vi "NanoRoute3D.vi"(2 "Incoming Handle":i32) -> ()   [LabVIEW 2012]
uses:
  <vilib>/Utility/inputDevices.llb/keyboardAcquire.vi
  Madlib.dll
panel:
  out "fit graph once":bool
  out "Type Descriptor":i16[](array[numeric])
  out "Saved Route":T1
  in  "Tab Control":T2(tab)
  in  "include 6":bool=TRUE
  in  "include 5":bool=TRUE
  in  "include 4":bool=TRUE
  in  "include 3":bool=TRUE
  in  "include 2":bool=TRUE
  in  "include 1":bool=TRUE
  in  "stop":bool
  out "Firmware Profile":i16
  out "Firmware Version 2":i16
  out "Product ID (in hex) 2":string
  out "DAC resolution (bits)":i16
  out "ADC resolution (bits)":i16
  out "Dll Version":i16
  out "Dll Revision":i16
  out "ADC Freq (ms)":dbl format="%.4f"
  out "DAC Freq (ms)":dbl format="%.4f"
  out "X axis":bool
  out "Y axis":bool
  out "Z axis":bool
  out "Aux axis":bool
  out "X Calibration 2":dbl caption="Calibration (um)" format="%.3f"
  out "Y Calibration 2":dbl format="%.3f"
  out "Z Calibration 2":dbl format="%.3f"
  out "Aux Calibration 2":dbl format="%.3f"
  out "Serial # 2":i32
  in  "handleIndex":i32(ring)
  out "DeviceLoaded":bool
  in  "include 7":bool
  in  "include 8":bool
  in  "include 9":bool
  in  "include 10":bool
  in  "Remove All":bool
  in  "Set All":bool
  in  "SaveDeviceData":bool
  out "Device Data":string
  in  "Initialize/Release USB":bool
  in  "include 11":bool=TRUE
  in  "include 12":bool=TRUE
  in  "include 13":bool=TRUE
  in  "include 14":bool=TRUE
  in  "Run backwards":bool
  in  "Relative Start":bool
  in  "gamepad":bool
  out "LivePosition":enum32{"disable", "enable"}(tab)
  out "X-Axis":dbl format="%.4f"
  out "Y-Axis":dbl format="%.4f"
  out "Z-Axis":dbl format="%.4f"
  in  "Command X":bool
  in  "Command Y":bool
  in  "Command Z":bool
  in  "X command":dbl format="%#.4f"
  in  "Z command":dbl format="%#_4f"
  in  "Y command":dbl format="%#.4f"
  out "Scanning Indicator":bool
  in  "LivePosition":bool
  in  "um":dbl
  in  "(ms)":dbl=100.0 min=0.033
  in  "Path Units":u8(ring) items=["ms", "dpts"]
  in  "Load":bool
  in  "SAVE":bool
  out "Custom Scans":T3(tab)
  in  "Pixel dwell":u32
  in  "Begin Raster":bool
  in  "Pixel":u32(ring)=1 items=["X axis"=1, "Y axis"=2, "Z axis"=3]
  in  "Line":u32(ring)=2 items=["X axis"=1, "Y axis"=2, "Z axis"=3, "Do Nothing"=4]
  in  "Frame":u32(ring)=3 items=["X axis"=1, "Y axis"=2, "Z axis"=3, "Do Nothing"=4]
  in  "Pixel delay":u32
  in  "End of Line delay":u32
  in  "Frame delay":u32
  out "Est. R.S. time":dbl format="%<%H:%M:%S>t"
  in  "Mirror motion on return?":bool=TRUE
  in  "Start of Line delay":u32
  in  "RaScAdvanced":bool
  out "Custom.name 2":string
  out "Custom.name 3":string
  in  "Ignore":bool
  in  "A/D Rate\n16-bit":dbl=2.0 min=0.033
  in  "A/D Rate\n20-bit":dbl(ring)=1.0 items=[".267ms"=0.267, ".5ms"=0.5, "1ms"=1.0, "2ms"=2.0, "10ms"=10.0, "17ms"=17.0, "20ms"=20.0]
  in  "Template":u16(ring) items=["Standard", "Single Axis Scan", "Multi-Axis Scan", "Raster Scan", "Custom Scan 1", "Custom Scan 2"]
  in  "Clear Graph":bool
  in  "WF\nAcq.":bool=TRUE
  in  "Run All Routes":bool
  out "Paths in Z Route:":u16
  out "Paths in Y Route:":u16
  in  "Axis":u32(ring)=1 items=["X axis"=1, "Y axis"=2, "Z axis"=3]
  out "Points in Route":i32
  out "Points in Current Path":i32
  in  "function:":string="sin(x)"
  out "Time to Command Route (ms):":dbl
  in  "Load Route":bool
  in  "Save Route":bool
  out "Paths in X Route:":u16
  in  "Reset":bool
  in  "Run Route":bool
  in  "Current #:":u16
  in  "DeletePath":bool
  in  "AddPath":bool
  in  "PrevPoint":bool
  in  "NextPoint":bool
  in  "Path Type":u16(ring) items=["Remain at", "Ramp to", "Apply Point Func:", "Apply Time Func:", "Custom Path 1", "Custom Path 2"]
  in  "offset":dbl[](array[numeric])
  out "Route Graph":cluster{dbl[], dbl[]}[](graph)=[{[0.0], [0.0]}, {[0.0, 1.0, 2.0, 3.0, 4.0, 5.0, 6.0, 7.0, 8.0, 9.0, 10.0, 11.0, 12.0, 13.0, 14.0, 15.0, 16.0, 17.0, 18.0, 19.0, 20.0, 21.0, 22.0, 23.0, 24.0, 25.0, 26.0, 27.0, 28.0, 29.0, 30.0, 31.0, 32.0, 33.0, 34.0, 35.0, 36.0, 37.0, 38.0, 39.0, 40.0, 41.0, 42.0, 43.0, 44.0, 45.0, 46.0, 47.0, 48.0, 49.0], [0.0, 0.0, 0.0, 0.0, 0.0, 0.0, 0.0, 0.0, 0.0, 0.0, 0.0, 0.0, 0.0, 0.0, 0.0, 0.0, 0.0, 0.0, 0.0, 0.0, 0.0, 0.0, 0.0, 0.0, 0.0, 0.0, 0.0, 0.0, 0.0, 0.0, 0.0, 0.0, 0.0, 0.0, 0.0, 0.0, 0.0, 0.0, 0.0, 0.0, 0.0, 0.0, 0.0, 0.0, 0.0, 0.0, 0.0, 0.0, 0.0, 0.0]}, {[], []}, {[], []}, {[], []}, {[], []}, {[], []}]
  in  "View Start of Scan ISS Commands":bool caption="View End of Scan ISS Commands"
  in  "Adv ISS Control":bool
  out "ISS pre-post config.":enum32{"Basic", "Adv. Start", "Adv. End"}(tab)
  in  "Start:Pixel":bool
  in  "Start:Line":bool
  in  "Start:Frame":bool
  in  "Start:Aux":bool
  in  "End:Pixel":bool
  in  "End:Line":bool
  in  "End:Frame":bool
  in  "End:Aux":bool
  in  "Start:Pixel:Order":enum16{"1st", "2nd", "3rd", "4th"}(ring)
  in  "Start:Line:Order":enum16{"1st", "2nd", "3rd", "4th"}(ring)=enum."2nd"
  in  "Start:Frame:Order":enum16{"1st", "2nd", "3rd", "4th"}(ring)=enum."3rd"
  in  "Start:Aux:Order":enum16{"1st", "2nd", "3rd", "4th"}(ring)=enum."4th"
  in  "End:Pixel:Order":enum16{"1st", "2nd", "3rd", "4th"}(ring)
  in  "End:Line:Order":enum16{"1st", "2nd", "3rd", "4th"}(ring)=enum."2nd"
  in  "End:Frame:Order":enum16{"1st", "2nd", "3rd", "4th"}(ring)=enum."3rd"
  in  "End:Aux:Order":enum16{"1st", "2nd", "3rd", "4th"}(ring)=enum."4th"
  out "ISSAdv Start":dbl
  in  "AuxStartAdv 11":bool=TRUE
  in  "AuxStartAdv 10":bool=TRUE
  in  "AuxStartAdv 9":bool=TRUE
  in  "AuxStartAdv 8":bool=TRUE
  in  "AuxStartAdv 7":bool=TRUE
  in  "AuxStartAdv 6":bool=TRUE
  in  "AuxStartAdv 5":bool=TRUE
  in  "AuxStartAdv 4":bool=TRUE
  in  "AuxStartAdv 3":bool=TRUE
  in  "AuxStartAdv 2":bool=TRUE
  in  "AuxStartAdv 1":bool=TRUE
  in  "FrameStartAdv 11":bool=TRUE
  in  "FrameStartAdv 10":bool=TRUE
  in  "FrameStartAdv 9":bool=TRUE
  in  "FrameStartAdv 8":bool=TRUE
  in  "FrameStartAdv 7":bool=TRUE
  in  "FrameStartAdv 6":bool=TRUE
  in  "FrameStartAdv 5":bool=TRUE
  in  "FrameStartAdv 4":bool=TRUE
  in  "FrameStartAdv 3":bool=TRUE
  in  "FrameStartAdv 2":bool=TRUE
  in  "FrameStartAdv 1":bool=TRUE
  in  "LineStartAdv 11":bool=TRUE
  in  "LineStartAdv 10":bool=TRUE
  in  "LineStartAdv 9":bool=TRUE
  in  "LineStartAdv 8":bool=TRUE
  in  "LineStartAdv 7":bool=TRUE
  in  "LineStartAdv 6":bool=TRUE
  in  "LineStartAdv 5":bool=TRUE
  in  "LineStartAdv 4":bool=TRUE
  in  "LineStartAdv 3":bool=TRUE
  in  "LineStartAdv 2":bool=TRUE
  in  "LineStartAdv 1":bool
  in  "PixStartAdv 11":bool=TRUE
  in  "PixStartAdv 10":bool=TRUE
  in  "PixStartAdv 9":bool=TRUE
  in  "PixStartAdv 8":bool=TRUE
  in  "PixStartAdv 7":bool=TRUE
  in  "PixStartAdv 6":bool=TRUE
  in  "PixStartAdv 5":bool=TRUE
  in  "PixStartAdv 4":bool=TRUE
  in  "PixStartAdv 3":bool=TRUE
  in  "PixStartAdv 2":bool=TRUE
  in  "PixStartAdv 1":bool=TRUE
  in  "ISS msStart 11":dbl
  in  "ISS msStart 10":dbl
  in  "ISS msStart 9":dbl
  in  "ISS msStart 8":dbl
  in  "ISS msStart 7":dbl
  in  "ISS msStart 6":dbl
  in  "ISS msStart 5":dbl
  in  "ISS msStart 4":dbl
  in  "ISS msStart 3":dbl
  in  "ISS msStart 2":dbl
  in  "ISS msStart 1":dbl
  in  "ISS msEnd 1":dbl
  in  "ISS msEnd 2":dbl
  in  "ISS msEnd 3":dbl
  in  "ISS msEnd 4":dbl
  in  "ISS msEnd 5":dbl
  in  "ISS msEnd 6":dbl
  in  "ISS msEnd 7":dbl
  in  "ISS msEnd 8":dbl
  in  "ISS msEnd 9":dbl
  in  "ISS msEnd 10":dbl
  in  "ISS msEnd 11":dbl
  in  "PixEndAdv 1":bool=TRUE
  in  "PixEndAdv 2":bool=TRUE
  in  "PixEndAdv 3":bool=TRUE
  in  "PixEndAdv 4":bool=TRUE
  in  "PixEndAdv 5":bool=TRUE
  in  "PixEndAdv 6":bool=TRUE
  in  "PixEndAdv 7":bool=TRUE
  in  "PixEndAdv 8":bool=TRUE
  in  "PixEndAdv 9":bool=TRUE
  in  "PixEndAdv 10":bool=TRUE
  in  "PixEndAdv 11":bool=TRUE
  in  "LineEndAdv 1":bool
  in  "LineEndAdv 2":bool=TRUE
  in  "LineEndAdv 3":bool=TRUE
  in  "LineEndAdv 4":bool=TRUE
  in  "LineEndAdv 5":bool=TRUE
  in  "LineEndAdv 6":bool=TRUE
  in  "LineEndAdv 7":bool=TRUE
  in  "LineEndAdv 8":bool=TRUE
  in  "LineEndAdv 9":bool=TRUE
  in  "LineEndAdv 10":bool=TRUE
  in  "LineEndAdv 11":bool=TRUE
  in  "FrameEndAdv 1":bool=TRUE
  in  "FrameEndAdv 2":bool=TRUE
  in  "FrameEndAdv 3":bool=TRUE
  in  "FrameEndAdv 4":bool=TRUE
  in  "FrameEndAdv 5":bool=TRUE
  in  "FrameEndAdv 6":bool=TRUE
  in  "FrameEndAdv 7":bool=TRUE
  in  "FrameEndAdv 8":bool=TRUE
  in  "FrameEndAdv 9":bool=TRUE
  in  "FrameEndAdv 10":bool=TRUE
  in  "FrameEndAdv 11":bool=TRUE
  in  "AuxEndAdv 1":bool=TRUE
  in  "AuxEndAdv 2":bool=TRUE
  in  "AuxEndAdv 3":bool=TRUE
  in  "AuxEndAdv 4":bool=TRUE
  in  "AuxEndAdv 5":bool=TRUE
  in  "AuxEndAdv 6":bool=TRUE
  in  "AuxEndAdv 7":bool=TRUE
  in  "AuxEndAdv 8":bool=TRUE
  in  "AuxEndAdv 9":bool=TRUE
  in  "AuxEndAdv 10":bool=TRUE
  in  "AuxEndAdv 11":bool=TRUE
  in  "PulseAux":bool
  in  "PulseFrame":bool
  in  "PulseLine":bool
  in  "LineRestore":bool
  in  "AuxRestore":bool
  in  "LinePol":enum16{"Low", "High"}(ring)
  in  "LinePulse":enum16{"Low to High", "High to Low"}(ring)
  in  "LineBindAxis":T4(ring)
  in  "FramePol":enum16{"Low", "High"}(ring)
  in  "FramePulse":enum16{"Low to High", "High to Low"}(ring)
  in  "FrameBindAxis":T4(ring)
  in  "FrameRestore":bool
  in  "AuxPol":enum16{"Low", "High"}(ring)
  in  "AuxPulse":enum16{"Low to High", "High to Low"}(ring)
  in  "AuxBindAxis":T4(ring)
  in  "PulsePix":bool
  in  "PixBindAxis":T4(ring)
  in  "PixPulse":enum16{"Low to High", "High to Low"}(ring)
  in  "ISSReset":bool
  in  "PixRestore":bool
  in  "ISSConfirm":bool
  in  "PixPol":enum16{"Low", "High"}(ring)
  in  "Export DAC":bool
  in  "Export ADC":bool
  in  "Now Showing":u32(ring) items=["Individual Route Scan", "Run All Routes Scan", "Raster Scan", "Custom 1", "Custom 2"]
  in  "Back Remove":u32(slide) step=1 scale=0.0..100.0
  in  "FrontRemove":u32(slide) step=1 scale=0.0..100.0
  in  "Y-Axis Display":u8(ring)=2 items=["Point by Point", "Time in milliseconds", "Axis: X Position", "Axis: Y Position", "Axis: Z Position"]
  in  "Legend Visible":bool
  in  "Interpolation?":bool=TRUE
  in  "Visible?":bool=TRUE
  in  "X-Axis Display":u8(ring) items=["Point by Point", "Time in milliseconds", "Axis: X Position", "Axis: Y Position", "Axis: Z Position"]
  in  "Active Plot":u32(ring) items=["ADC values (Sensor)", "DAC values (Command)"]
  out "Image Graph":cluster{dbl[], dbl[]}[](graph)
  # "Device Information"
  # "Version 2.01"
  # "Device Information"
  # "Data will be saved to a text file in the following format:"
  # "Load/Release USB(s)"
  # "Include/Disinclude All:"
  # "Available Devices:"
  # "Calibration (um)"
  # "Nano-Route  3D"
  # "®"
  # "VI State Control"
  # "Generate/Run Route"
  # "Scan Type"
  # "Device Settings"
  # "A/D\nRate"
  # "(ms)"
  # "New Path"
  # "over an interval of ..."
  # "dpts"
  # "Path Creation"
  # "Copy/Paste Route"
  # "Route Settings"
  # "Relative start"
  # "Nano-Drive Live Position"
  # "Gamepad"
  # "Check box at left to enable live position updates. This feature may interfere with your ISS settings"
  # "um"
  # "um"
  # "um"
  # "um"
  # "um"
  # "um"
  # "Raster Scan"
  # "ms"
  # "ms"
  # "ms"
  # "ms"
  # "ms"
  # "ISS Configuration"
  # "Pixel Clock"
  # "Line Clock"
  # "Frame Clock"
  # "Auxilary Clock"
  # "Polarity:"
  # "Polarity:"
  # "Polarity:"
  # "Polarity:"
  # "Pulse:"
  # "Pulse:"
  # "Pulse:"
  # "Pulse:"
  # "Bind Clock to Axis:"
  # "Bind Clock to Axis:"
  # "Bind Clock to Axis:"
  # "Bind Clock to Axis:"
  # "* Only one clock can be bound to an axis or event. Binding a second clock\n    replaces the first with the second (Nano-Route   3D prevents this action)."
  # "®"
  # "Confirm/Reset \nISS Configuration:"
  # "* Changes made here take no effect until confirmed."
  # "* Binding a Clock to an Axis will result in the suspension of \"Nano-Drive Live\n  Position\" reads."
  # "Programmatic ISS Control"
  # "Pulse Individual \nISS Clocks:"
  # "* Pulsing will reset Clock to Low polarity."
  # "Pulse clock before beginning each scan."
  # "Pulse clock at the end of each scan."
  # "Pixel clock"
  # "Pixel clock"
  # "Line clock"
  # "Line clock"
  # "Frame clock"
  # "Frame clock"
  # "Aux clock"
  # "Aux clock"
  # "milliseconds"
  # "ms"
  # "pixel clock"
  # "Start\nof \nScan"
  # "line clock"
  # "frame clock"
  # "aux clock"
  # "milliseconds"
  # "pixel clock"
  # "End\nof \nScan"
  # "line clock"
  # "frame clock"
  # "aux clock"
  # "Crop Data-\n Points From \n  Start/End"
  # "Plot to Edit:"
  # "X-Axis Repr.:"
  # "Graph Options"
  # "Plot Options"
  # "Now Showing:"
  # "Y-Axis Repr.:"
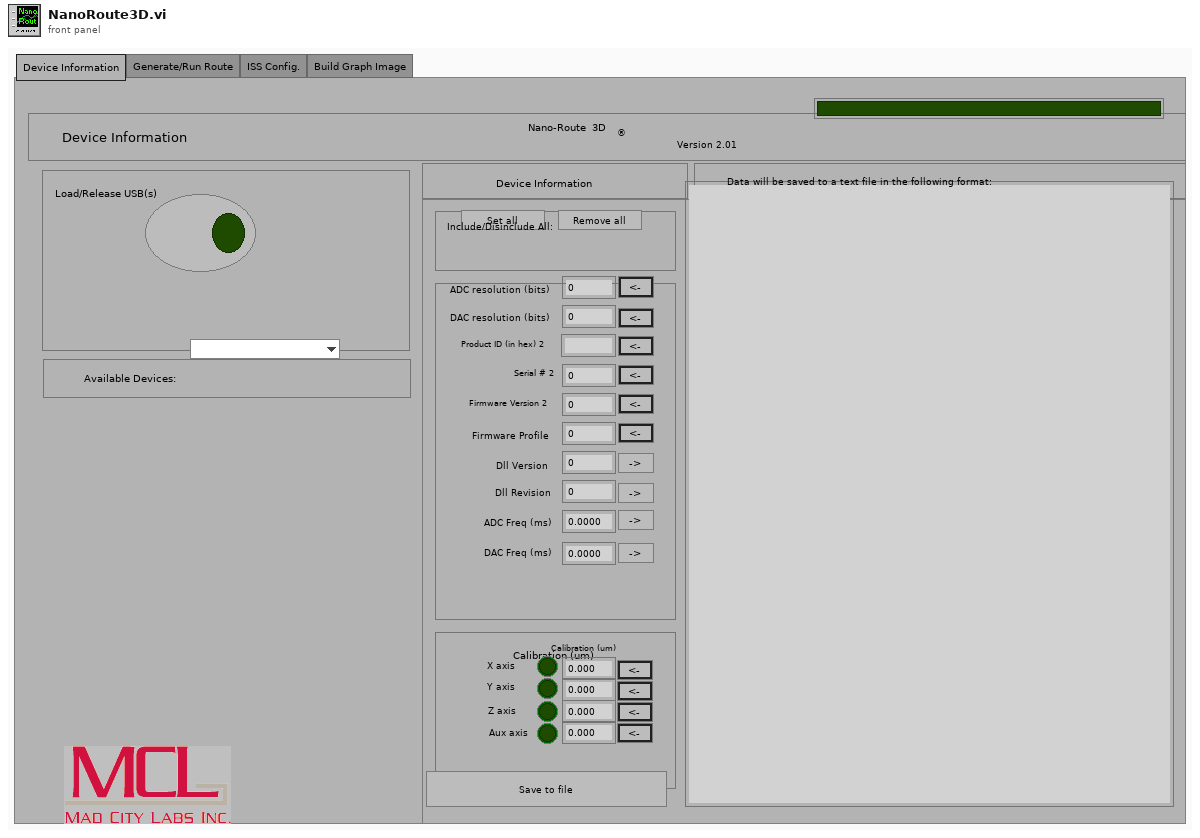
[diagram p1: front panel]
types:
  T1 = cluster{"t":cluster{dbl[], dbl[], i32[], u16[]}, "Current Path #:":u16, "# of Paths in Route:":u16}
  T2 = enum32{"Device Information", "Generate/Run Route", "ISS Config.", "Build Graph Image"}
  T3 = enum32{"Empty", "Raster Scan", "Custom 1", "Custom 2"}
  T4 = enum16{"Unbound", "X Axis", "Y Axis", "Z Axis", "Auxilary", "Waveform Read", "Waveform Write"}
  T5 = cluster{"Pixel delay":u32, "End of Line delay":u32, "Start of Line delay":u32, "Frame delay":u32, "Pixel dwell":u32}
  T6 = cluster{"X axis":bool, "Y axis":bool, "Z axis":bool}
  T7 = cluster{"Incoming Handle":i32, "Axis":u32, "A/D Rate\n16-bit 2":dbl}
  T8 = cluster{"RaSc16bitReadRate IN":dbl, "RaSc16bitWriteRate IN":dbl, "RaSc20bitWriteRate IN":dbl, "RaSc20bitReadRate IN":dbl, "Pixel uses Waveform Acquisition IN":bool, "RaSc16bit#ofReads IN":u32}
  T9 = cluster{"ISSReset":bool, "ISS Confirmed Options":cluster{"clock (1=Pixel)":i32, "Pixel Polarity":enum16{"Low", "High"}, "Pixel Pulse":enum16{"Low to High", "High to Low"}, "Pixel Bind":enum16{"Unbound", "X Axis", "Y Axis", "Z Axis", "Auxilary", "Waveform Read", "Waveform Write"}}, "ISS Confirmed Options":cluster{"clock (1=Pixel)":i32, "Pixel Polarity":enum16{"Low", "High"}, "Pixel Pulse":enum16{"Low to High", "High to Low"}, "Pixel Bind":enum16{"Unbound", "X Axis", "Y Axis", "Z Axis", "Auxilary", "Waveform Read", "Waveform Write"}}, "ISS Confirmed Options":cluster{"clock (1=Pixel)":i32, "Pixel Polarity":enum16{"Low", "High"}, "Pixel Pulse":enum16{"Low to High", "High to Low"}, "Pixel Bind":enum16{"Unbound", "X Axis", "Y Axis", "Z Axis", "Auxilary", "Waveform Read", "Waveform Write"}}, "ISS Confirmed Options":cluster{"clock (1=Pixel)":i32, "Pixel Polarity":enum16{"Low", "High"}, "Pixel Pulse":enum16{"Low to High", "High to Low"}, "Pixel Bind":enum16{"Unbound", "X Axis", "Y Axis", "Z Axis", "Auxilary", "Waveform Read", "Waveform Write"}}}
  T10 = cluster{"Custom 1 Read Arrays":cluster{"Z Read":cluster{dbl[], dbl[]}, "Y Read":cluster{i32[], dbl[]}, "Z Read":cluster{i32[], dbl[]}}, "Custom 1 Read Arrays":cluster{"Z Read":cluster{dbl[], dbl[]}, "Y Read":cluster{i32[], dbl[]}, "Z Read":cluster{i32[], dbl[]}}}
  T11 = cluster{"handlesListIndex":i32, "listOfHandlist":i32[], "sizeOfHandlesList":i32}
  T12 = cluster{"Read":cluster{dbl[], "Waveform Read":dbl[]}, "Read":cluster{dbl[], "Waveform Read":dbl[]}, "Read":cluster{dbl[], "Waveform Read":dbl[]}}
  T13 = enum16{"0", "1", "2", "3", "4", "5", "6", "7", "8", "9", "A", "B", "C", "D", "E", "F", "G", "H", "I", "J", "K", "L", "M", "N", "O", "P", "Q", "R", "S", "T", "U", "V", "W", "X", "Y", "Z", "F1", "F2", "F3", "F4", "F5", "F6", "F7", "F8", "F9", "F10", "F11", "F12", "F13", "F14", "F15", "ADD", "BACK", "BACKSLASH", "CAPITAL", "COMMA", "DECIMAL", "DELETE", "DIVIDE", "DOWN", "END", "EQUALS", "ESCAPE", "GRAVE (`)", "HOME", "INSERT", "LBRACKET", "LCONTROL", "LEFT", "L ALT", "LSHIFT", "LWIN", "MINUS", "MULTIPLY", "NEXT", "NUMLOCK", "NUMPAD_0", "NUMPAD_1", "NUMPAD_2", "NUMPAD_3", "NUMPAD_4", "NUMPAD_5", "NUMPAD_6", "NUMPAD_7", "NUMPAD_8", "NUMPAD_9", "PAUSE", "PERIOD", "PRIOR (PG UP)", "RBRACKET", "RCONTROL", "RETURN", "RIGHT", "R ALT", "RSHIFT", "RWIN", "SCROLL", "SEMICOLON", "SLASH", "SPACE", "SUBTRACT", "TAB", "UP", "ENTER (num pad)", "' (quote)"}[]
  T14 = cluster{cluster{dbl[], dbl[]}, cluster{dbl[], dbl[]}, cluster{dbl[], dbl[]}}
  T15 = cluster{string, cluster{"ADC resolution (bits)":i16, "DAC resolution (bits)":i16, "Product ID (in hex)":string, "Firmware Version":i16, "Firmware Profile":i16, "Dll Version":i16, "X axis":bool, "Y axis":bool, "Z axis":bool, "Aux axis":bool, "X Calibration":dbl, "Y Calibration":dbl, "Z Calibration":dbl, "Aux Calibration":dbl, "Dll Revision":i16, "ADC Freq (ms)":dbl, "DAC Freq (ms)":dbl, "Serial #":i32}, "X Calibration":dbl, "Y Calibration":dbl, "Z Calibration":dbl, bool}
  T16 = enum32{"Device Information", "Generate/Run Route", "ISS Config.", "Rptblty Test", "Build Graph Image", "Set Gain/Offset"}
  T17 = cluster{cluster{refnum<vi>[], refnum<vi>[], refnum<vi>[], refnum<vi>[], refnum<vi>[]}, cluster{refnum<vi>[], refnum<vi>[], refnum<vi>[], refnum<vi>[], refnum<vi>[]}}
  T18 = cluster{cluster{"Start:Pixel":bool, "Start:Line":bool, "Start:Frame":bool, "Start:Aux":bool, "End:Pixel":bool, "End:Line":bool, "End:Frame":bool, "End:Aux":bool}, refnum<vi>[], cluster{"Start:Pixel:Order":enum16{"1st", "2nd", "3rd", "4th"}, "Start:Line:Order":enum16{"1st", "2nd", "3rd", "4th"}, "Start:Frame:Order":enum16{"1st", "2nd", "3rd", "4th"}, "Start:Aux:Order":enum16{"1st", "2nd", "3rd", "4th"}, "End:Pixel:Order":enum16{"1st", "2nd", "3rd", "4th"}, "End:Line:Order":enum16{"1st", "2nd", "3rd", "4th"}, "End:Frame:Order":enum16{"1st", "2nd", "3rd", "4th"}, "End:Aux:Order":enum16{"1st", "2nd", "3rd", "4th"}}, refnum<vi>[]}
  T19 = enum32{"Device Information", "Generate/Run Route", "ISS Config.", "Build Graph Image", "Set Gain/Offset"}
  T20 = enum16{"0", "1", "2", "3", "4", "5", "6", "7", "8", "9", "A", "B", "C", "D", "E", "F", "G", "H", "I", "J", "K", "L", "M", "N", "O", "P", "Q", "R", "S", "T", "U", "V", "W", "X", "Y", "Z", "F1", "F2", "F3", "F4", "F5", "F6", "F7", "F8", "F9", "F10", "F11", "F12", "F13", "F14", "F15", "ADD", "BACK", "BACKSLASH", "CAPITAL", "COMMA", "DECIMAL", "DELETE", "DIVIDE", "DOWN", "END", "EQUALS", "ESCAPE", "GRAVE (`)", "HOME", "INSERT", "LBRACKET", "LCONTROL", "LEFT", "L ALT", "LSHIFT", "LWIN", "MINUS", "MULTIPLY", "NEXT", "NUMLOCK", "NUMPAD_0", "NUMPAD_1", "NUMPAD_2", "NUMPAD_3", "NUMPAD_4", "NUMPAD_5", "NUMPAD_6", "NUMPAD_7", "NUMPAD_8", "NUMPAD_9", "PAUSE", "PERIOD", "PRIOR (PG UP)", "RBRACKET", "RCONTROL", "RETURN", "RIGHT", "R ALT", "RSHIFT", "RWIN", "SCROLL", "SEMICOLON", "SLASH", "SPACE", "SUBTRACT", "TAB", "UP", "ENTER (num pad)", "' (quote)"}
  T21 = cluster{"Z":cluster{dbl[], dbl[], i32[], u16[]}, "Y":cluster{dbl[], dbl[], i32[], u16[]}, "X":cluster{dbl[], dbl[], i32[], u16[]}}
  T22 = cluster{"Route Graph":refnum<vi>, "Axis":refnum<vi>, "A/D Rate\n16-bit":refnum<vi>}
  T23 = cluster{"Xaxis":cluster{dbl[], "command":dbl[], i32[], u16[]}, "Yaxis":cluster{dbl[], "command":dbl[], i32[], u16[]}, "Zaxis":cluster{dbl[], "command":dbl[], i32[], u16[]}}
  T24 = cluster{"Current #:":u16, "Path Type":u16, "um":dbl, "function:":string, i32[], dbl, dbl[], dbl, "A/D Rate\n16-bit":dbl, "Path Units":u8}
  T25 = cluster{"Start:Pixel:Order":enum16{"1st", "2nd", "3rd", "4th"}, "Start:Line:Order":enum16{"1st", "2nd", "3rd", "4th"}, "Start:Frame:Order":enum16{"1st", "2nd", "3rd", "4th"}, "Start:Aux:Order":enum16{"1st", "2nd", "3rd", "4th"}, "End:Pixel:Order":enum16{"1st", "2nd", "3rd", "4th"}, "End:Line:Order":enum16{"1st", "2nd", "3rd", "4th"}, "End:Frame:Order":enum16{"1st", "2nd", "3rd", "4th"}, "End:Aux:Order":enum16{"1st", "2nd", "3rd", "4th"}}
  T26 = cluster{"Start:Pixel":bool, "Start:Line":bool, "Start:Frame":bool, "Start:Aux":bool, "End:Pixel":bool, "End:Line":bool, "End:Frame":bool, "End:Aux":bool}
  T27 = cluster{refnum<vi>[], refnum<vi>[], refnum<vi>[], refnum<vi>[], refnum<vi>[]}
  T28 = cluster{"Template":u16, "Template":u16, "pulse template":bool}
  T29 = cluster{"clock (1=Pixel)":i32, "Pixel Polarity":enum16{"Low", "High"}, "Pixel Pulse":enum16{"Low to High", "High to Low"}, "Pixel Bind":enum16{"Unbound", "X Axis", "Y Axis", "Z Axis", "Auxilary", "Waveform Read", "Waveform Write"}}
  T30 = cluster{"ADC resolution (bits) ":refnum<vi>, "DAC resolution (bits) ":refnum<vi>, "Product ID (in hex) 2":refnum<vi>, "Firmware Version 2":refnum<vi>, "Firmware Profile ":refnum<vi>, "Dll Version ":refnum<vi>, "X axis":refnum<vi>, "Y axis":refnum<vi>, "Z axis":refnum<vi>, "Aux axis":refnum<vi>, "X Calibration 2":refnum<vi>, "Y Calibration 2":refnum<vi>, "Z Calibration 2":refnum<vi>, "Aux Calibration 2":refnum<vi>, "Dll Revision ":refnum<vi>, "ADC Freq (ms) ":refnum<vi>, "DAC Freq (ms) ":refnum<vi>, "Serial # 2":refnum<vi>}
  T31 = cluster{"ADC resolution (bits)":i16, "DAC resolution (bits)":i16, "Product ID (in hex)":string, "Firmware Version":i16, "Firmware Profile":i16, "Dll Version":i16, "X axis":bool, "Y axis":bool, "Z axis":bool, "Aux axis":bool, "X Calibration":dbl, "Y Calibration":dbl, "Z Calibration":dbl, "Aux Calibration":dbl, "Dll Revision":i16, "ADC Freq (ms)":dbl, "DAC Freq (ms)":dbl, "Serial #":i32}
  T32 = cluster{"handleIndex":i32, "listOfHandlist":i32[], "sizeOfHandlesList":i32}
  T33 = cluster{"include 1":refnum<vi>, "include 2":refnum<vi>, "include 3":refnum<vi>, "include 4":refnum<vi>, "include 5":refnum<vi>, "include 6":refnum<vi>, "include 7":refnum<vi>, "include 8":refnum<vi>, "include 9":refnum<vi>, "include 10":refnum<vi>, "include 11":refnum<vi>, "include 12":refnum<vi>, "include 13":refnum<vi>, "include 14":refnum<vi>}
  T34 = cluster{"Mirror motion on return?":bool, "Raster Scan Advanced Options OUT":cluster{"RaSc16bitReadRate IN":dbl, "RaSc16bitWriteRate IN":dbl, "RaSc20bitWriteRate IN":dbl, "RaSc20bitReadRate IN":dbl, "Pixel uses Waveform Acquisition IN":bool, "RaSc16bit#ofReads IN":u32}, "RasterAxisConfig":cluster{"Pixel":u32, "Line":u32, "Frame":u32}, "RasterDelays":cluster{"Pixel delay":u32, "End of Line delay":u32, "Start of Line delay":u32, "Frame delay":u32, "Pixel dwell":u32}}
  T35 = cluster{"Relative Start":bool, "offset":dbl, "Incoming Handle":i32}
  T36 = cluster{"Setup WF Read":cluster{"axis":u32, "datapoints":u32, "milliseconds":dbl}, "Setup WF Load":cluster{"axis":u32, "datapoints":i32, "milliseconds":dbl, "waveform":dbl[]}, cluster{"axis":u32, "# of reads":u32, "array buffer":dbl[]}}
  T37 = cluster{"Text":string, "Device Info OUT":cluster{"ADC resolution (bits)":i16, "DAC resolution (bits)":i16, "Product ID (in hex)":string, "Firmware Version":i16, "Firmware Profile":i16, "Dll Version":i16, "X axis":bool, "Y axis":bool, "Z axis":bool, "Aux axis":bool, "X Calibration":dbl, "Y Calibration":dbl, "Z Calibration":dbl, "Aux Calibration":dbl, "Dll Revision":i16, "ADC Freq (ms)":dbl, "DAC Freq (ms)":dbl, "Serial #":i32}, "X Calibration":dbl, "Y Calibration":dbl, "Z Calibration":dbl, "20bit":bool}
  T38 = cluster{"Pixel Route":dbl[], "Line Route":dbl[], "Frame Route":dbl[]}
  T39 = cluster{cluster{"Text":string, "Device Info OUT":cluster{"ADC resolution (bits)":i16, "DAC resolution (bits)":i16, "Product ID (in hex)":string, "Firmware Version":i16, "Firmware Profile":i16, "Dll Version":i16, "X axis":bool, "Y axis":bool, "Z axis":bool, "Aux axis":bool, "X Calibration":dbl, "Y Calibration":dbl, "Z Calibration":dbl, "Aux Calibration":dbl, "Dll Revision":i16, "ADC Freq (ms)":dbl, "DAC Freq (ms)":dbl, "Serial #":i32}, "X Calibration":dbl, "Y Calibration":dbl, "Z Calibration":dbl, "20bit":bool}, "Read":cluster{dbl[], "Waveform Read":dbl[]}, cluster{dbl[], dbl[]}, "Read":cluster{dbl[], "Waveform Read":dbl[]}}
  T40 = cluster{"Pixel Read Arrays":dbl[][], "Line Read Arrays":dbl[][], "Frame Read Arrays":dbl[][]}
  T41 = cluster{"Current #:":refnum<vi>, "Axis":refnum<vi>, "Paths in X Route:":refnum<vi>, "Paths in Y Route:":refnum<vi>, "Paths in Z Route:":refnum<vi>}
  T42 = cluster{"Saved Route":refnum<vi>, "Axis":refnum<vi>, "Current #:":refnum<vi>, "Paths in X Route:":refnum<vi>, "Paths in Y Route:":refnum<vi>, "Paths in Z Route:":refnum<vi>}
  T43 = cluster{"string":string, "string":string, "string":string, "string":string, "string":string, "string":string, "string":string, "string":string, "string":string}
  T44 = cluster{"Z":cluster{dbl[], dbl[], i32[], u16[]}, "Y":cluster{dbl[], dbl[], i32[], u16[]}, "X":cluster{dbl[], dbl[], i32[], u16[]}, "Incoming Handle":i32, "Axis":u32, "A/D Rate\n16-bit 2":dbl, "A/D Rate\n16-bit":dbl, "Paths in X Route:":u16, "Paths in Y Route:":u16, "Paths in Z Route:":u16, "Template":u16, cluster{"ISSReset":bool, "ISS Confirmed Options":cluster{"clock (1=Pixel)":i32, "Pixel Polarity":enum16{"Low", "High"}, "Pixel Pulse":enum16{"Low to High", "High to Low"}, "Pixel Bind":enum16{"Unbound", "X Axis", "Y Axis", "Z Axis", "Auxilary", "Waveform Read", "Waveform Write"}}, "ISS Confirmed Options":cluster{"clock (1=Pixel)":i32, "Pixel Polarity":enum16{"Low", "High"}, "Pixel Pulse":enum16{"Low to High", "High to Low"}, "Pixel Bind":enum16{"Unbound", "X Axis", "Y Axis", "Z Axis", "Auxilary", "Waveform Read", "Waveform Write"}}, "ISS Confirmed Options":cluster{"clock (1=Pixel)":i32, "Pixel Polarity":enum16{"Low", "High"}, "Pixel Pulse":enum16{"Low to High", "High to Low"}, "Pixel Bind":enum16{"Unbound", "X Axis", "Y Axis", "Z Axis", "Auxilary", "Waveform Read", "Waveform Write"}}, "ISS Confirmed Options":cluster{"clock (1=Pixel)":i32, "Pixel Polarity":enum16{"Low", "High"}, "Pixel Pulse":enum16{"Low to High", "High to Low"}, "Pixel Bind":enum16{"Unbound", "X Axis", "Y Axis", "Z Axis", "Auxilary", "Waveform Read", "Waveform Write"}}}, cluster{"Mirror motion on return?":bool, "Raster Scan Advanced Options OUT":cluster{"RaSc16bitReadRate IN":dbl, "RaSc16bitWriteRate IN":dbl, "RaSc20bitWriteRate IN":dbl, "RaSc20bitReadRate IN":dbl, "Pixel uses Waveform Acquisition IN":bool, "RaSc16bit#ofReads IN":u32}, "RasterAxisConfig":cluster{"Pixel":u32, "Line":u32, "Frame":u32}, "RasterDelays":cluster{"Pixel delay":u32, "End of Line delay":u32, "Start of Line delay":u32, "Frame delay":u32, "Pixel dwell":u32}}}
  T45 = cluster{"clock (1=Pixel)":i32, "Pixel Polarity":enum16{"Low", "High"}, "Pixel Pulse":enum16{"Low to High", "High to Low"}, "Pixel Bind":enum16{"Unbound", "X Axis", "Y Axis", "Z Axis", "Auxilary", "Waveform Read", "Waveform Write"}}[]
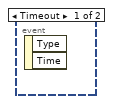
[diagram p3: hidden frame]
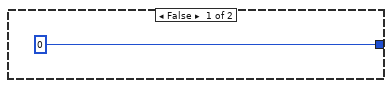
[diagram p4: hidden frame]
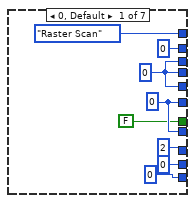
[diagram p9: hidden frame]
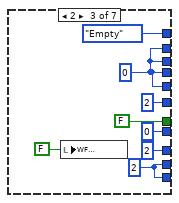
[diagram p10: hidden frame]
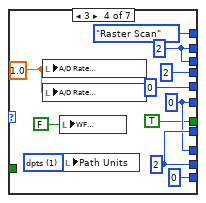
[diagram p11: hidden frame]
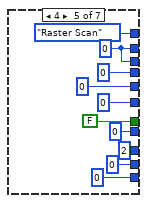
[diagram p12: hidden frame]
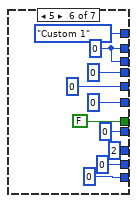
[diagram p13: hidden frame]
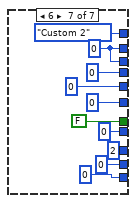
[diagram p14: hidden frame]
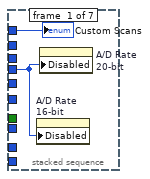
[diagram p15: hidden frame]
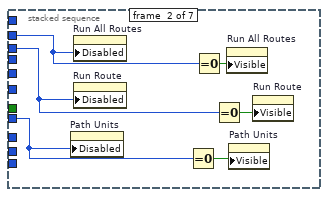
[diagram p16: hidden frame]
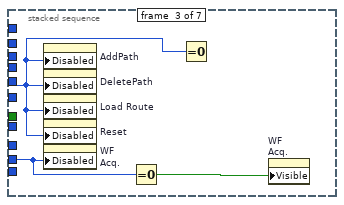
[diagram p17: hidden frame]
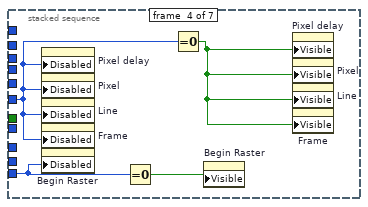
[diagram p18: hidden frame]
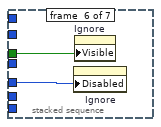
[diagram p19: hidden frame]
diagram:
  w1 = dbl[] []  # TimeStampArray
  w2 = T5 {"Pixel delay"=0, "End of Line delay"=0, "Start of Line delay"=0, "Frame delay"=0, "Pixel dwell"=0}  # RasterDelays
  w3 = cluster{"Pixel":u32, "Line":u32, "Frame":u32} {"Pixel"=0, "Line"=0, "Frame"=0}  # RasterAxisConfig
  w39 = TRUE  # pulse template
  w43 = T10 {"Custom 1 Read Arrays"={"Z Read"={[], []}, "Y Read"={[], []}, "Z Read"={[], []}}, "Custom 1 Read Arrays"={"Z Read"={[], []}, "Y Read"={[], []}, "Z Read"={[], []}}}  # Custom Graph Data
  w44 = cluster{dbl[], dbl[], i32[], u16[]} {[], [], [], []} ("t")
  w40 = u8 0  # Template
  w48 = T13 [enum."0"] items=["0", "1", "2", "3", "4", "5", "6", "7", "8", "9", "A", "B", "C", "D", "E", "F", "G", "H", "I", "J", "K", "L", "M", "N", "O", "P", "Q", "R", "S", "T", "U", "V", "W", "X", "Y", "Z", "F1", "F2", "F3", "F4", "F5", "F6", "F7", "F8", "F9", "F10", "F11", "F12", "F13", "F14", "F15", "ADD", "BACK", "BACKSLASH", "CAPITAL", "COMMA", "DECIMAL", "DELETE", "DIVIDE", "DOWN", "END", "EQUALS", "ESCAPE", "GRAVE (`)", "HOME", "INSERT", "LBRACKET", "LCONTROL", "LEFT", "L ALT", "LSHIFT", "LWIN", "MINUS", "MULTIPLY", "NEXT", "NUMLOCK", "NUMPAD_0", "NUMPAD_1", "NUMPAD_2", "NUMPAD_3", "NUMPAD_4", "NUMPAD_5", "NUMPAD_6", "NUMPAD_7", "NUMPAD_8", "NUMPAD_9", "PAUSE", "PERIOD", "PRIOR (PG UP)", "RBRACKET", "RCONTROL", "RETURN", "RIGHT", "R ALT", "RSHIFT", "RWIN", "SCROLL", "SEMICOLON", "SLASH", "SPACE", "SUBTRACT", "TAB", "UP", "ENTER (num pad)", "' (quote)"] ("keys pressed")
  w52 = u16 0 ("Current Point:")
  w56 = FALSE  # Device Loaded?
  # "y"
  # "z"
  # "x"
  # "Raster Scan image"
  # "AD Rate"
  # "axis"
  n1 = event shown="[1] Panel Close?" {
    selector: _ -> [_ _]
    dyn-events: _ -> [_ _]
    timeout: -1 -> [_ _]
    event Timeout {
      n2 = event-data() -> ()  [unwired: 3 out]
    }
    event Panel Close? {
      n3 = event-data() -> ()  [unwired: 5 out]
      n4 = flat-sequence {
        frame #0 {
          # "Stop Sequence"
          n5 = for {
            N: 20 -> [_]
            n6 = dll-call lib="C:/Users/Labview/Desktop/64-bit VIs/Madlib.dll" fn="MCL_ReleaseAllHandles"() -> ()  [unwired: 3 in, 3 out]
          }
        }
        frame #1 {
          n7 = Quit LabVIEW(quit? (T)=TRUE ("stop? (T)")) -> ()
        }
        frame #2 {
          n8 = Stop(stop? (T)=TRUE) -> ()
        }
      }
      n9 = event-data("Discard?"=TRUE) -> ()  [unwired: 1 in, 1 out]
    }
  }
  n10 = Current VI's Path() -> (path=w35:path)
  n11 = Bundle("include 1"="include 1", "include 2"="include 2", "include 3"="include 3", "include 4"="include 4", "include 5"="include 5", "include 6"="include 6", "include 7"="include 7", "include 8"="include 8", "include 9"="include 9", "include 10"="include 10", "include 11"="include 11", "include 12"="include 12", "include 13"="include 13", "include 14"="include 14") -> ()  [unwired: 2 out]
  n12 = Strip Path(path=w35) -> (stripped path=w34:path)  [unwired: 1 out]
  n13 = flat-sequence {
    frame #0 {
      n14 = property on="handleIndex" class="Ring (strict)"("Strings []"=string[] [" "]) -> ()  [unwired: 2 in, 2 out]
    }
    frame #1 {
      n15 = local write "handleIndex"(u16 0 ("Paths in Z Route:")) -> ()
    }
  }
  n16 = Strip Path(path=w34) -> (stripped path=w33:path, name=w32:string)
  n17 = String To Path(string=w32) -> (path=w31:path)
  n18 = call <vilib>:"Get File Extension.vi"("file"=w31) -> ("lowercase file extension"=w29:string)  [unwired: 1 in, 9 out]
  n19 = local write "Paths in X Route:"(w52) -> ()
  n20 = local write "Paths in Y Route:"(w52) -> ()
  n21 = local write "Paths in Z Route:"(w52) -> ()
  n22 = local write "Current #:"(w52) -> ()
  n23 = control-ref of="stop"() -> (w26:refnum<vi>)
  n24 = Equal?(x=w29, y="exe" ("lowercase file extension")) -> (x = y?=w28:bool)
  n25 = Get Date/Time In Seconds() -> (seconds since 1Jan1904=w24:timestamp)
  n26 = Build Path(base path=w33, name or relative path="visettings.txt") -> ()  [unwired: 1 out]
  n27 = Not(x=w28) -> (.not. x?=w27:bool)
  n28 = property on="offset" class="Arr (strict)"("Value"=dbl[] [0.0, 0.0, 0.0] ("offset")) -> ()  [unwired: 2 in, 2 out]
  n29 = Build Array(w24) -> (w23:timestamp[])
  n30 = property on="Property Node" class="Bool (strict)"(reference=w26, "Visible"=w27) -> ()  [unwired: 1 in, 2 out]
  n31 = property class="Bool (strict)"(reference=w26, "Value"=FALSE) -> ()  [unwired: 1 in, 2 out]
  n32 = call <vilib>:"Intialize Keyboard.vi"() -> ("device ID"=w49:refnum<k1>)  [unwired: 1 in, 10 out]
  n33 = Bundle("Template"=w40, "pulse template"=w39) -> (w38:cluster{"Template":u8, "pulse template":bool})  [unwired: 1 out]
  n34 = while {
    shift-right: [w138] -> _
    shift-left: w56 -> [w329]
    shift-right: [w75] -> _
    shift-left: T15 {"", {"ADC resolution (bits)"=0, "DAC resolution (bits)"=0, "Product ID (in hex)"="", "Firmware Version"=0, "Firmware Profile"=0, "Dll Version"=0, "X axis"=FALSE, "Y axis"=FALSE, "Z axis"=FALSE, "Aux axis"=FALSE, "X Calibration"=0.0, "Y Calibration"=0.0, "Z Calibration"=0.0, "Aux Calibration"=0.0, "Dll Revision"=0, "ADC Freq (ms)"=0.0, "DAC Freq (ms)"=0.0, "Serial #"=0}, "X Calibration"=0.0, "Y Calibration"=0.0, "Z Calibration"=0.0, FALSE} -> [w74]
    shift-right: [w77] -> _
    shift-left: "Incoming Handle" -> [w76]
    shift-right: [w349] -> _
    shift-left: w44 -> [w393]
    shift-right: [w135] -> _
    shift-left: T12 {"Read"={[], "Waveform Read"=[]}, "Read"={[], "Waveform Read"=[]}, "Read"={[], "Waveform Read"=[]}} -> [w154]
    shift-right: [w137] -> _
    shift-left: T12 {"Read"={[], "Waveform Read"=[]}, "Read"={[], "Waveform Read"=[]}, "Read"={[], "Waveform Read"=[]}} -> [w367]
    shift-right: [w136] -> _
    shift-left: cluster{dbl[], dbl[]} {[], []} -> [w280]
    shift-right: [w350] -> _
    shift-left: w44 -> [w392]
    shift-right: [w351] -> _
    shift-left: w44 -> [w391]
    shift-right: [w348] -> _
    shift-left: _ -> [w283]
    shift-right: [w83] -> _
    shift-left: T14 {{[], []}, {[], []}, {[], []}} ("All Route Reads") -> [w84]
    shift-right: [w347] -> _
    shift-left: _ -> [w282]
    shift-right: [w89] -> _
    shift-left: cluster{dbl[], dbl[], dbl[]} {[], [], []} -> [w268]
    tunnel: w49 -> [w379]
    shift-right: [w86] -> _
    shift-left: w48 -> [w87]
    shift-right: [w164] -> _
    shift-left: w38 -> [w173]
    shift-right: [w226] -> _
    shift-left: T9 {"ISSReset"=FALSE, "ISS Confirmed Options"={"clock (1=Pixel)"=0, "Pixel Polarity"=enum."Low", "Pixel Pulse"=enum."Low to High", "Pixel Bind"=enum."Unbound"}, "ISS Confirmed Options"={"clock (1=Pixel)"=0, "Pixel Polarity"=enum."Low", "Pixel Pulse"=enum."Low to High", "Pixel Bind"=enum."Unbound"}, "ISS Confirmed Options"={"clock (1=Pixel)"=0, "Pixel Polarity"=enum."Low", "Pixel Pulse"=enum."Low to High", "Pixel Bind"=enum."Unbound"}, "ISS Confirmed Options"={"clock (1=Pixel)"=0, "Pixel Polarity"=enum."Low", "Pixel Pulse"=enum."Low to High", "Pixel Bind"=enum."Unbound"}} -> [w146]
    shift-right: [w324] -> _
    shift-left: T11 {"handlesListIndex"=0, "listOfHandlist"=[], "sizeOfHandlesList"=0} -> [w322]
    shift-right: [w139] -> _
    shift-left: T8 {"RaSc16bitReadRate IN"=1.0, "RaSc16bitWriteRate IN"=1.0, "RaSc20bitWriteRate IN"=1.0, "RaSc20bitReadRate IN"=5.0, "Pixel uses Waveform Acquisition IN"=FALSE, "RaSc16bit#ofReads IN"=0} ("Raster Scan Advanced Options OUT") -> [w85]
    shift-right: [w88] -> _
    shift-left: w43 -> [w88]
    shift-right: [w160] -> _
    shift-left: _ -> [w159]
    tunnel: ["stop"] -> w6
    shift-right: [w129] -> _
    shift-left: w23 -> [w131]
    shift-right: [w81] -> _
    shift-left: T7 {"Incoming Handle"=0, "Axis"=0, "A/D Rate\n16-bit 2"=0.0} ("Axis Info") -> [w80]
    shift-right: [w79] -> _
    shift-left: T6 {"X axis"=FALSE, "Y axis"=FALSE, "Z axis"=FALSE} ("Active Axes") -> [w78]
    shift-right: ["Axis"] -> _
    shift-left: _ -> [w72]
    shift-right: [w71] -> _
    shift-left: w3 -> [w69]
    shift-right: [w70] -> _
    shift-left: w2 -> [w68]
    shift-right: [w65] -> _
    shift-left: w1 -> [w63]
    stop <- "stop" stop-if-true
    w340 = u8 4 items=["Custom", "Single Axis Scan", "Multi-Axis Scan", "Raster Scan", "Load MCL Scan"] ("Template")
    w371 = T20."LCONTROL" ("keyType 3")
    # "gamepad"
    # "save/load"
    # "live position control"
    # "raster scan"
    # "scan"
    # "devices"
    # "keyboard"
    # "Template"
    # "ISS"
    # "Graph"
    # "Route"
    # "if\n   -  Template was set to \"Load MCL Scan\"\n   && Template feedback is not the same\n   || Load button pressed\n  then\n   -Load MCL Scan"
    # "scan time"
    n35 = case shown="3" w72 {
      tunnel: w367 -> [w1462 w1464 w1466]
      tunnel: [w1461 w1463 w1465] -> w90
      frame 2 {
        n36 = Unbundle(w1462) -> ("Read"=w1461:cluster{dbl[], "Waveform Read":dbl[]})  [unwired: 2 out]
      }
      frame 3 {
        n37 = Unbundle(w1464) -> ("Read"=w1463:cluster{dbl[], "Waveform Read":dbl[]})  [unwired: 2 out]
      }
      frame 1, Default {
        n38 = Unbundle(w1466) -> ("Read"=w1465:cluster{dbl[], "Waveform Read":dbl[]})  [unwired: 2 out]
      }
    }
    n39 = Wait Until Next ms Multiple(millisecond multiple=u32 5) -> ()  [unwired: 1 out]
    n40 = case shown="1, Default" w72 {
      tunnel: w154 -> [w1468 w1470 w1472]
      tunnel: [w1467 w1469 w1471] -> w234
      frame 2 {
        n41 = Unbundle(w1468) -> ("Read"=w1467:cluster{dbl[], "Waveform Read":dbl[]})  [unwired: 2 out]
      }
      frame 3 {
        n42 = Unbundle(w1470) -> ("Read"=w1469:cluster{dbl[], "Waveform Read":dbl[]})  [unwired: 2 out]
      }
      frame 1, Default {
        n43 = Unbundle(w1472) -> ("Read"=w1471:cluster{dbl[], "Waveform Read":dbl[]})  [unwired: 2 out]
      }
    }
    n44 = Equal?(x="Tab Control", y=u32 2 ("max queue size (-1, unlimited)")) -> (x = y?=w320:bool)
    n45 = Equal?(x="Tab Control", y=u32 3) -> (x = y?=w321:bool)
    n46 = Equal?(x="Tab Control", y=u32 1 ("max queue size (-1, unlimited)")) -> (x = y?=w319:bool)
    n47 = local write "Scanning Indicator"(FALSE ("Scanning Indicator")) -> ()
    n48 = case shown="1, Default" w72 {
      tunnel: [w1616 w1617 w1618] -> w272
      tunnel: w393 -> [w1616 _ _]
      tunnel: w392 -> [_ w1617 _]
      tunnel: w391 -> [_ _ w1618]
      frame 1, Default {
      }
      frame 2 {
      }
      frame 3 {
      }
    }
    n49 = Not(x=w329) -> (.not. x?=w416:bool)
    n50 = Compound Arithmetic op=OR(w319, w320, w321) -> (w318:bool)
    n51 = Not(x="Initialize/Release USB") -> (.not. x?=w331:bool)
    n52 = And(x=w416, y=w318) -> (x .and. y?=w417:bool)
    n53 = And(x=w329, y=w331) -> (x .and. y?=w413:bool)
    n54 = call-poly <vilib>:"Acquire Input Data.vi"("device ID"=w379) -> ("keys pressed"=w86:T13)  [unwired: 1 in, 17 out]
    n55 = Bundle("Z"=w391, "Y"=w392, "X"=w393) -> (w267:T21)  [unwired: 1 out]
    n56 = case shown="True" w417 {
      frame False {
      }
      frame True {
        n57 = local write "Tab Control"(u32 0 ("max queue size (-1, unlimited)")) -> ()
      }
    }
    n58 = Not(x=w329) -> (.not. x?=w328:bool)
    n59 = case shown="3" w72 {
      tunnel: [w1613 w1614 w1615] -> w270
      frame 1, Default {
        n60 = local read "Paths in X Route:"() -> (w1613:u16)
      }
      frame 2 {
        n61 = local read "Paths in Y Route:"() -> (w1614:u16)
      }
      frame 3 {
        n62 = local read "Paths in Z Route:"() -> (w1615:u16)
      }
    }
    n63 = And(x=w328, y="Initialize/Release USB") -> (x .and. y?=w419:bool)
    n64 = And(x=w329, y="Initialize/Release USB") -> (x .and. y?=w323:bool)
    n65 = Index Array(array=w87, index=0) -> (element=w372:T20)
    n66 = Index Array(array=w86, index=0) -> (element=w375:T20)
    n67 = case shown="True" w413 {
      tunnel: w76 -> [w1636 _]
      tunnel: [w1636 0 ("Incoming Handle")] -> w412
      frame False {
      }
      frame True {
        n68 = flat-sequence {
          frame #0 {
            n69 = property on="handleIndex" class="Ring (strict)"("Strings []"=string[] [" "]) -> ()  [unwired: 2 in, 2 out]
          }
          frame #1 {
            w1639 = 0 items=[" "] ("handleIndex")
            n70 = local write "handleIndex"(w1639) -> ()
          }
        }
        n71 = dll-call lib="C:/Users/Labview/Desktop/64-bit VIs/Madlib.dll" fn="MCL_ReleaseAllHandles"() -> ()  [unwired: 3 in, 3 out]
      }
    }
    n72 = Equal?(x=w372, y=w371) -> (x = y?=w373:bool)
    n73 = Equal?(x=w375, y=w371) -> (x = y?=w374:bool)
    n74 = Unbundle(w74) -> ("20bit"=w261:bool)  [unwired: 5 out]
    n75 = case shown="True" w373 {
      tunnel: w374 -> [_ w1478]
      tunnel: [FALSE ("x = y?") FALSE ("x = y?")] -> w370
      frame False {
      }
      frame True {
        n76 = case shown="False" w1478 {
          frame True {
            n77 = stacked-sequence {
              frame #0 {
                n78 = property on="Route Graph" class="XYGraph (strict)"("Active Plot"=u32 2) -> ()  [unwired: 2 in, 2 out]
              }
              frame #1 {
                n79 = property on="Route Graph" class="XYGraph (strict)"("Plot.Plot Interpolation"=u8 0) -> ()  [unwired: 2 in, 2 out]
                n80 = property on="Route Graph" class="XYGraph (strict)"("Plot.Point Style"=u8 2) -> ()  [unwired: 2 in, 2 out]
              }
              frame #2 {
                n81 = property on="Route Graph" class="XYGraph (strict)"("Active Plot"=u32 1) -> ()  [unwired: 2 in, 2 out]
              }
              frame #3 {
                n82 = property on="Route Graph" class="XYGraph (strict)"("Plot.Plot Interpolation"=u8 0) -> ()  [unwired: 2 in, 2 out]
                n83 = property on="Route Graph" class="XYGraph (strict)"("Plot.Point Style"=u8 2) -> ()  [unwired: 2 in, 2 out]
              }
            }
          }
          frame False {
            n84 = stacked-sequence {
              frame #0 {
                n85 = property on="Route Graph" class="XYGraph (strict)"("Active Plot"=u32 2) -> ()  [unwired: 2 in, 2 out]
              }
              frame #1 {
                n86 = property on="Route Graph" class="XYGraph (strict)"("Plot.Plot Interpolation"=u8 2) -> ()  [unwired: 2 in, 2 out]
                n87 = property on="Route Graph" class="XYGraph (strict)"("Plot.Point Style"=u8 0) -> ()  [unwired: 2 in, 2 out]
              }
              frame #2 {
                n88 = property on="Route Graph" class="XYGraph (strict)"("Active Plot"=u32 1) -> ()  [unwired: 2 in, 2 out]
              }
              frame #3 {
                n89 = property on="Route Graph" class="XYGraph (strict)"("Plot.Plot Interpolation"=u8 2) -> ()  [unwired: 2 in, 2 out]
                n90 = property on="Route Graph" class="XYGraph (strict)"("Plot.Point Style"=u8 0) -> ()  [unwired: 2 in, 2 out]
              }
            }
          }
        }
      }
    }
    n91 = flat-sequence {
      tunnel: w261 -> [w1104]
      tunnel: w76 -> [w1098]
      tunnel: w179 -> [w1105]
      tunnel: w267 -> [w1106]
      tunnel: w269 -> [w1107]
      tunnel: w234 -> [w1108]
      tunnel: w84 -> [w1109]
      tunnel: w90 -> [w1110]
      tunnel: [w1110] -> w221
      tunnel: ["The A/D rate must be greater \nthan or equal to 6ms to scan all \nroutes. Correct this error and \ntry again." ("message")] -> w220
      tunnel: [w1109] -> w219
      tunnel: [w1108] -> w218
      tunnel: [w1107] -> w217
      tunnel: [w1106] -> w216
      tunnel: [w1105] -> w215
      tunnel: [w1098] -> w214
      tunnel: [w1104] -> w213
      tunnel: w192 -> [w1099]
      tunnel: [w1099] -> w206
      tunnel: ["WF\nAcq."] -> w198
      tunnel: [w1095] -> w197
      tunnel: ["Run All Routes"] -> w196
      tunnel: w184 -> [w1096]
      tunnel: [w1097] -> w187
      tunnel: [w1096] -> w185
      tunnel: w159 -> [w1094]
      tunnel: [w1094] -> w158
      tunnel: w146 -> [w1093]
      tunnel: [w1093] -> w145
      tunnel: w131 -> [w1092]
      tunnel: [w1092] -> w132
      tunnel: ["Run backwards"] -> w118
      tunnel: w63 -> [w1089]
      tunnel: [w1089] -> w64
      tunnel: w221 -> [w1142]
      tunnel: w220 -> [w1141]
      tunnel: w219 -> [w1140]
      tunnel: w218 -> [w1139]
      tunnel: w217 -> [w1118]
      tunnel: w216 -> [w1138]
      tunnel: w215 -> [w1137]
      tunnel: w214 -> [w1119]
      tunnel: w213 -> [w1129]
      tunnel: [w1136] -> w212
      tunnel: [w1135] -> w211
      tunnel: [w1134] -> w210
      tunnel: [w1133] -> w209
      tunnel: [w1119] -> w208
      tunnel: [w1128] -> w207
      tunnel: w206 -> [w1128]
      tunnel: w198 -> [w1127]
      tunnel: w197 -> [w1121]
      tunnel: w196 -> [w1126]
      tunnel: [w1121] -> w195
      tunnel: [w1125] -> w188
      tunnel: w187 -> [w1125]
      tunnel: [w1124] -> w186
      tunnel: w185 -> [w1124]
      tunnel: [w1122] -> w161
      tunnel: w158 -> [_]
      tunnel: w145 -> [w1116]
      tunnel: [w1116] -> w144
      tunnel: [w1115] -> w133
      tunnel: w132 -> [w1120]
      tunnel: w118 -> [w1114]
      tunnel: [w1112] -> w66
      tunnel: w64 -> [w1111]
      tunnel: [w1144] -> w274
      tunnel: [w1153] -> w276
      tunnel: [w1154] -> w277
      tunnel: [w1155] -> w278
      tunnel: [w1156] -> w279
      tunnel: w212 -> [w1156]
      tunnel: w211 -> [w1155]
      tunnel: w210 -> [w1154]
      tunnel: w209 -> [w1153]
      tunnel: w208 -> [w1150]
      tunnel: w207 -> [w1151]
      tunnel: w195 -> [w1144]
      tunnel: w188 -> [w1149]
      tunnel: w186 -> [w1148]
      tunnel: w161 -> [w1147]
      tunnel: [w1147] -> w160
      tunnel: w144 -> [w1146]
      tunnel: w133 -> [w1145]
      tunnel: [w1145] -> w130
      tunnel: w66 -> [w1143]
      tunnel: [w1143] -> w65
      frame #0 {
        n92 = Or(x="Run Route", y="Run All Routes") -> (x .or. y?=w1095:bool)
        n93 = local read "Adv ISS Control"() -> (w1097:bool)
        n94 = call "_nr_ISSprepost.vi"("Before Scan"=TRUE ("End:Aux"), "ISS pre-post Use Advanced"=w1097, "ISS pre-post"=w1099, "Handle"=w1098, "ISS pre-post Advanced Config"=w1096, "ISS Info"=w1093, "Enable"=w1095) -> ()  [unwired: 2 out]
        n95 = local write "Scanning Indicator"(w1095) -> ()
      }
      frame #1 {
        # "BEGIN SCANNING"
        n96 = control-ref of="Route Graph"() -> (w1132:refnum<vi>)
        n97 = control-ref of="A/D Rate\n16-bit"() -> (w1130:refnum<vi>)
        n98 = control-ref of="Axis"() -> (w1131:refnum<vi>)
        n99 = Bundle("Route Graph"=w1132, "Axis"=w1131, "A/D Rate\n16-bit"=w1130) -> (w1117:T22)  [unwired: 1 out]
        n100 = call "_nr_ScanRoute.vi"("PathGen References"=w1117, "20bit"=w1129, 2:"Read"=w1139, "WF Acq."=w1127, "New Route"=w1118, "run"=w1121, "Run All Routes"=w1126, "All Routes"=w1138, "All Route Reads"=w1140, "A/D Rate 16-bit"=w1137, "message"=w1141, "Incoming Handle"=w1119, 12:"Read"=w1142, "Relative Start"="Relative Start", "time_of_scan"=w1120, "TimeStampArray"=w1111, "offset"="offset", "Run backwards"=w1114) -> ("time_of_scan"=w1115:timestamp[], "Old Read"=w1136:cluster{dbl[], "Waveform Read":dbl[]}, "All Route Reads"=w1135:T14, "Recent Read"=w1134:cluster{dbl[], "Waveform Read":dbl[]}, "TimeStampArray"=w1112:dbl[], "error"=w1133:i32, "All Routes last read"=w1122:T23)  [unwired: 3 out]
      }
      frame #2 {
        n101 = call "_nr_ISSprepost.vi"("Before Scan"=FALSE ("End:Aux"), "ISS pre-post Use Advanced"=w1149, "ISS pre-post"=w1151, "Handle"=w1150, "ISS pre-post Advanced Config"=w1148, "ISS Info"=w1146, "Enable"=w1144) -> ()  [unwired: 2 out]
      }
    }
    n102 = flat-sequence {
      tunnel: w146 -> [w1184]
      tunnel: w298 -> [w1192]
      tunnel: w80 -> [w1190]
      tunnel: w110 -> [w1193]
      tunnel: w268 -> [w1194]
      tunnel: [w1194] -> w205
      tunnel: [w1193] -> w204
      tunnel: [w1190] -> w203
      tunnel: [w1192] -> w202
      tunnel: [w1184] -> w201
      tunnel: w192 -> [w1189]
      tunnel: ["Begin Raster"] -> w193
      tunnel: w184 -> [w1185]
      tunnel: [w1202] -> w297
      tunnel: [w1201] -> w296
      tunnel: [w1199] -> w295
      tunnel: [w1197] -> w294
      tunnel: [w1196] -> w257
      tunnel: w205 -> [w1202]
      tunnel: w204 -> [w1201]
      tunnel: w203 -> [w1198]
      tunnel: w202 -> [w1200]
      tunnel: w201 -> [w1196]
      tunnel: [w1195] -> w194
      tunnel: w193 -> [w1195]
      tunnel: ["Pixel delay"] -> w383
      tunnel: ["End of Line delay"] -> w382
      tunnel: ["Frame delay"] -> w381
      tunnel: ["Start of Line delay"] -> w380
      tunnel: [w1204] -> w141
      tunnel: ["RaScAdvanced"] -> w317
      tunnel: ["Pixel"] -> w288
      tunnel: ["Line"] -> w287
      tunnel: ["Frame"] -> w286
      tunnel: ["Mirror motion on return?"] -> w223
      tunnel: [w1209] -> w299
      tunnel: [w1208] -> w300
      tunnel: [w1206] -> w156
      tunnel: [w1207] -> w231
      tunnel: w297 -> [w1209]
      tunnel: w296 -> [w1208]
      tunnel: w295 -> [w1207]
      tunnel: w294 -> [w1206]
      tunnel: w85 -> [w1205]
      tunnel: [w1205] -> w178
      tunnel: w257 -> [_]
      tunnel: w194 -> [w1204]
      tunnel: ["Pixel dwell"] -> w142
      frame #0 {
        n103 = Unbundle(w1190) -> ("Incoming Handle"=w1188:i32)  [unwired: 2 out]
        n104 = local read "Adv ISS Control"() -> (w1186:bool)
        n105 = call "_nr_ISSprepost.vi"("Before Scan"=TRUE ("End:Aux"), "ISS pre-post Use Advanced"=w1186, "ISS pre-post"=w1189, "Handle"=w1188, "ISS pre-post Advanced Config"=w1185, "ISS Info"=w1184, "Enable"="Begin Raster") -> ()  [unwired: 2 out]
      }
      frame #1 {
        # "ISS Info\n\n--------------------------------\n--------------------------------"
        # "--------------------------------\n--------------------------------\nAxis Info"
        # "--------------------------------\n--------------------------------\n\nRoutes"
        # "Device Info\n\n--------------------------------\n--------------------------------"
        # "--------------------------------\n--------------------------------\n\nRaster Image"
        n106 = Unbundle(w1200) -> ("20bit"=w1199:bool)  [unwired: 5 out]
        n107 = Unbundle(w1198) -> ("Incoming Handle"=w1197:i32)  [unwired: 2 out]
      }
      frame #2 {
        # "--------------------------------\n--------------------------------\n\nRaster Scan Options"
        n108 = local write "Scanning Indicator"(w1204) -> ()
      }
    }
    n109 = flat-sequence {
      tunnel: [w945] -> w397
      tunnel: [w944] -> w396
      tunnel: [w942] -> w395
      tunnel: [w935] -> w316
      tunnel: w272 -> [w934]
      tunnel: w270 -> [w933]
      tunnel: [w932] -> w265
      tunnel: ["Path Units"] -> w263
      tunnel: w261 -> [w930]
      tunnel: [w929] -> w260
      tunnel: [w928] -> w259
      tunnel: "Current #:" -> [w927]
      tunnel: [w926] -> w179
      frame #0 {
        # "INTERPRET PATH PARAMETERS"
        # "Define limits for cycling\nthrough Points"
        # "# of\npoints"
        n110 = Select(t="A/D Rate\n20-bit", s=w930, f="A/D Rate\n16-bit") -> (s? t:f=w936:dbl)
        n111 = Less?(x=w927, y=w933) -> (x < y?=w949:bool)
        n112 = Greater Than 0?(x=w927) -> (x > 0?=w951:bool)
        n113 = Not(x=w930) -> (.not. x?=w937:bool)
        n114 = And(x=w949, y="NextPoint") -> (x .and. y?=w950:bool)
        n115 = And(x=w951, y="PrevPoint") -> (x .and. y?=w952:bool)
        n116 = property on="A/D Rate\n20-bit" class="Ring (strict)"("Visible"=w930) -> ()  [unwired: 2 in, 2 out]
        n117 = property on="A/D Rate\n16-bit" class="DigNum (strict)"("Visible"=w937) -> ()  [unwired: 2 in, 2 out]
        n118 = Unbundle(w934) -> (w955:dbl[], w946:dbl[], w947:i32[], w954:u16[])
        n119 = Decrement(x=w927) -> (x-1=w956:u16)
        n120 = Increment(x=w927) -> (x+1=w957:u16)
        n121 = Or(x=w950, y=w952) -> (x .or. y?=w958:bool)
        n122 = stacked-sequence {
          seq-local: [w960 _ _] -> [_ w978 _]
          seq-local: [_ w972 _] -> [_ _ w1017]
          tunnel: [_ _ "um"] -> w942
          tunnel: [_ _ "(ms)"] -> w941
          tunnel: [_ _ w1019] -> w940
          tunnel: [_ _ w1014] -> w928
          tunnel: w950 -> [w964 _ _]
          tunnel: w952 -> [_ _ _]
          tunnel: w958 -> [w965 w979 _]
          tunnel: w957 -> [w963 _ _]
          tunnel: w956 -> [w962 _ _]
          tunnel: w927 -> [w961 _ _]
          tunnel: [w960 _ _] -> w929
          tunnel: w955 -> [_ w977 _]
          tunnel: w946 -> [_ w976 _]
          tunnel: w947 -> [_ w975 _]
          tunnel: w954 -> [_ w974 _]
          tunnel: [_ w973 _] -> w945
          tunnel: "Path Units" -> [_ _ w1018]
          tunnel: [_ _ w1017] -> w926
          tunnel: w936 -> [_ w971 _]
          tunnel: [_ _ w1012] -> w935
          frame #0 {
            n123 = case shown="True" w965 {
              tunnel: w964 -> [_ w970]
              tunnel: w963 -> [_ w969]
              tunnel: w962 -> [_ w968]
              tunnel: [w966 w967] -> w960
              tunnel: w961 -> [w966 _]
              frame False {
              }
              frame True {
                n124 = Select(t=w969, s=w970, f=w968) -> (s? t:f=w967:u16)
                n125 = local write "Current #:"(w967) -> ()
              }
            }
          }
          frame #1 {
            n126 = case shown="True" w979 {
              tunnel: w978 -> [w981 w996]
              tunnel: w977 -> [w985 w1002]
              tunnel: w976 -> [_ w1003]
              tunnel: w975 -> [w986 w998]
              tunnel: w974 -> [_ w997]
              tunnel: [w984 w1001] -> w973
              tunnel: [w980 w991] -> w972
              tunnel: w971 -> [w980 w991]
              frame False {
                n127 = for {
                  N: w981 -> [_]
                  tunnel: w986 -> [w988] mode=indexing
                  shift-right: [w990] -> w983
                  shift-left: 0 -> [w989]
                  tunnel: [w988] -> _
                  n128 = Add(x=w989, y=w988) -> (x+y=w990:i32)
                }
                n129 = Decrement(x=w983) -> (x-1=w982:i32)
                n130 = Index Array(array=w985, index=w982) -> (element=w984:dbl)
              }
              frame True {
                # "X pos"
                # "Total # of points"
                # "current point"
                n131 = for {
                  N: w996 -> [_]
                  tunnel: w998 -> [w1009] mode=indexing
                  shift-right: [w1011] -> w999
                  shift-left: 0 -> [w1010]
                  n132 = Add(x=w1010, y=w1009) -> (x+y=w1011:i32)
                }
                n133 = Index Array(array=w998, index=w996) -> (element=w993:i32)
                n134 = Equal To 0?(x=w993) -> (x = 0?=w994:bool)
                n135 = case shown="False" w994 {
                  tunnel: w993 -> [w1007 _]
                  tunnel: w991 -> [w1006 _]
                  tunnel: [w1005 10.0] -> w992
                  frame False {
                    n136 = Multiply(x=w1006, y=w1007) -> (x*y=w1005:dbl)
                  }
                  frame True {
                  }
                }
                n137 = Index Array "Index Array"(array=w997, index=w996) -> (element=w995:u16)
                n138 = Index Array "Index Array"(array=w1002, index=w999) -> (element=w1001:dbl)
                n139 = Index Array(array=w1003, index=w999) -> (element=w1004:dbl)
                n140 = local write "Path Type"(w995) -> ()
                n141 = local write "(ms)"(w992) -> ()
                n142 = local write "um"(w1004) -> ()
              }
            }
          }
          frame #2 {
            n143 = case shown="0, Default" w1018 {
              tunnel: w1017 -> [w1022 _]
              tunnel: [w1022 1.0 ("A/D\nRate")] -> w1019
              frame 0, Default {
              }
              frame 1 {
              }
            }
            n144 = Equal?(x=u8 10, y="Path Type") -> (x = y?=w1012:bool)
            n145 = Select(t=u8 2, s=w1012, f="Path Type") -> (s? t:f=w1014:u16)
          }
        }
        n146 = Bundle(w955, w946) -> (w932:cluster{dbl[], dbl[]})  [unwired: 1 out]
        n147 = Divide(x=w941, y=w940) -> (x/y=w943:dbl)
        n148 = Bundle("Current #:"=w929, "Path Type"=w928, "um"=w942, "function:"="function:", w947, w943, w946, w945, "A/D Rate\n16-bit"=w926, "Path Units"="Path Units") -> (w944:T24)  [unwired: 1 out]
      }
    }
    n149 = Equal?(x=T2."Build Graph Image" ("Tab Control"), y="Tab Control") -> (x = y?=w150:bool)
    n150 = case shown="True" w150 {
      tunnel: w268 -> [_ w430]
      tunnel: w84 -> [_ w429]
      tunnel: [u32 0 ("Now Showing") w428] -> w266
      tunnel: w88 -> [_ w427]
      tunnel: w179 -> [_ w426]
      tunnel: w159 -> [_ w425]
      tunnel: w154 -> [_ w424]
      tunnel: w131 -> [_ w422]
      tunnel: w63 -> [_ w421]
      frame False {
      }
      frame True {
        n151 = flat-sequence {
          tunnel: w430 -> [w447]
          tunnel: w429 -> [w446]
          tunnel: w427 -> [w444]
          tunnel: w426 -> [w443]
          tunnel: w425 -> [w442]
          tunnel: w424 -> [w441]
          tunnel: ["Now Showing"] -> w423
          tunnel: w422 -> [w432]
          tunnel: w421 -> [w431]
          tunnel: [w450] -> w428
          tunnel: w423 -> [w450]
          frame #0 {
            # "BUILD GRAPH IMAGE"
            n152 = control-ref of="Image Graph"() -> (w440:refnum<vi>)
            n153 = call "_nr_GraphImage.vi"("New Raster Image"=w447, "A/D Rate\n16-bit 2"=w443, "Now Showing"="Now Showing", "Recent Scans"=w441, "All Route Reads"=w446, "All Routes"=w442, "Back Remove"="Back Remove", "X-Axis Display"="X-Axis Display", "TimeStampArray"=w431, "FrontRemove"="FrontRemove", "Y-Axis Display"="Y-Axis Display", "Image Graph"=w440, "Export ADC"="Export ADC", "Custom Graph Data"=w444, "Export DAC"="Export DAC", "time_of_scan"=w432) -> ("Image Graph"=→"Image Graph":cluster{dbl[], dbl[]}[])  [unwired: 11 in]
          }
          frame #1 {
            w449 = u8 1  # Scale Fit
            n154 = local read "fit graph once"() -> (w448:bool)
            n155 = case shown="True" w448 {
              tunnel: w449 -> [_ w452]
              frame False {
              }
              frame True {
                n156 = property on="Image Graph" class="XYGraph (strict)"("YScale.ScaleFit"=w452, "XScale.ScaleFit"=w452) -> ()  [unwired: 2 in, 2 out]
                n157 = local write "fit graph once"(FALSE ("fit graph once")) -> ()
              }
            }
          }
        }
      }
    }
    n158 = control-ref of="X axis"() -> (w247:refnum<vi>)
    n159 = control-ref of="Y axis"() -> (w246:refnum<vi>)
    n160 = control-ref of="Z axis"() -> (w245:refnum<vi>)
    n161 = control-ref of="Aux axis"() -> (w244:refnum<vi>)
    n162 = Unbundle(w80) -> ("Incoming Handle"=w334:i32, "Axis"=w359:u32, "A/D Rate\n16-bit 2"=w358:dbl)
    n163 = control-ref of="ADC resolution (bits)"() -> (w253:refnum<vi>)
    n164 = control-ref of="DAC resolution (bits)"() -> (w252:refnum<vi>)
    n165 = control-ref of="Firmware Version 2"() -> (w250:refnum<vi>)
    n166 = control-ref of="Firmware Profile"() -> (w249:refnum<vi>)
    n167 = control-ref of="Dll Version"() -> (w248:refnum<vi>)
    n168 = control-ref of="Product ID (in hex) 2"() -> (w251:refnum<vi>)
    n169 = Unbundle(w173) -> ("Template"=w172:u16, "pulse template"=w170:bool)
    n170 = case shown="True" "Adv ISS Control" {
      tunnel: [w620 T18 {{"Start:Pixel"=FALSE, "Start:Line"=FALSE, "Start:Frame"=FALSE, "Start:Aux"=FALSE, "End:Pixel"=FALSE, "End:Line"=FALSE, "End:Frame"=FALSE, "End:Aux"=FALSE}, [], {"Start:Pixel:Order"=enum."1st", "Start:Line:Order"=enum."1st", "Start:Frame:Order"=enum."1st", "Start:Aux:Order"=enum."1st", "End:Pixel:Order"=enum."1st", "End:Line:Order"=enum."1st", "End:Frame:Order"=enum."1st", "End:Aux:Order"=enum."1st"}, []}] -> w192
      tunnel: [T17 {{[], [], [], [], []}, {[], [], [], [], []}} w722] -> w184
      frame False {
        n171 = property on="View Start of Scan ISS Commands" class="Bool (strict)"("Visible"=FALSE) -> ()  [unwired: 2 in, 2 out]
        n172 = local write "ISS pre-post config."(enum32{"Basic", "Adv. Start", "Adv. End"}."Basic" ("ISS pre-post config.")) -> ()
        n173 = control-ref of="Start:Pixel"() -> (w648:refnum<vi>)
        n174 = control-ref of="Start:Line"() -> (w647:refnum<vi>)
        n175 = control-ref of="Start:Frame"() -> (w646:refnum<vi>)
        n176 = control-ref of="Start:Aux"() -> (w645:refnum<vi>)
        n177 = control-ref of="End:Pixel"() -> (w644:refnum<vi>)
        n178 = control-ref of="End:Line"() -> (w643:refnum<vi>)
        n179 = control-ref of="End:Frame"() -> (w642:refnum<vi>)
        n180 = control-ref of="End:Aux"() -> (w641:refnum<vi>)
        n181 = Bundle("Start:Pixel:Order"="Start:Pixel:Order", "Start:Line:Order"="Start:Line:Order", "Start:Frame:Order"="Start:Frame:Order", "Start:Aux:Order"="Start:Aux:Order", "End:Pixel:Order"="End:Pixel:Order", "End:Line:Order"="End:Line:Order", "End:Frame:Order"="End:Frame:Order", "End:Aux:Order"="End:Aux:Order") -> (w626:T25)  [unwired: 1 out]
        n182 = Build Array(w648, w647, w646, w645, w644, w643, w642, w641) -> (w639:refnum<vi>[])
        n183 = control-ref of="Start:Pixel:Order"() -> (w630:refnum<vi>)
        n184 = control-ref of="Start:Line:Order"() -> (w622:refnum<vi>)
        n185 = control-ref of="Start:Frame:Order"() -> (w621:refnum<vi>)
        n186 = control-ref of="Start:Aux:Order"() -> (w629:refnum<vi>)
        n187 = control-ref of="End:Pixel:Order"() -> (w628:refnum<vi>)
        n188 = control-ref of="End:Line:Order"() -> (w627:refnum<vi>)
        n189 = control-ref of="End:Frame:Order"() -> (w631:refnum<vi>)
        n190 = control-ref of="End:Aux:Order"() -> (w632:refnum<vi>)
        n191 = Bundle("Start:Pixel"="Start:Pixel", "Start:Line"="Start:Line", "Start:Frame"="Start:Frame", "Start:Aux"="Start:Aux", "End:Pixel"="End:Pixel", "End:Line"="End:Line", "End:Frame"="End:Frame", "End:Aux"="End:Aux") -> (w640:T26)  [unwired: 1 out]
        n192 = Build Array(w630, w622, w621, w629, w628, w627, w631, w632) -> (w625:refnum<vi>[])
        n193 = Bundle(w640, w639, w626, w625) -> (w620:T18)  [unwired: 1 out]
        n194 = event shown="[1] \"Start:Pixel:Order\", \"Start:Line:Order\", \"Start:Frame:Order\", \"Start:Aux:Order\": Value Change" {
          selector: _ -> [_ _]
          dyn-events: _ -> [_ _]
          timeout: 1 -> [_ _]
          tunnel: w620 -> [_ w684]
          event Timeout {
            n195 = event-data() -> ()  [unwired: 3 out]
          }
          event "Start:Pixel:Order", "Start:Line:Order", "Start:Frame:Order", "Start:Aux:Order": Value Change {
            n196 = event-data() -> ("CtlRef"=w685:refnum<vi>, "OldVal"=w682:enum16{"1st", "2nd", "3rd", "4th"})  [unwired: 5 out]
            n197 = Unbundle(w684) -> (w683:refnum<vi>[])  [unwired: 3 out]
            n198 = while {
              tunnel: w685 -> [w696]
              tunnel: w683 -> [w695] mode=indexing
              tunnel: w682 -> [w686]
              i -> [w691]
              stop <- w688 stop-if-true
              n199 = Not Equal?(x=w696, y=w695) -> (x != y?=w694:bool)
              n200 = property class="Enum (strict)"(reference=w696) -> (reference out=w698:refnum<vi>, "Value"=w692:enum16{"1st", "2nd", "3rd", "4th"})  [unwired: 1 in, 1 out]
              n201 = property class="Enum (strict)"(reference=w695) -> (reference out=w697:refnum<vi>, "Value"=w693:enum16{"1st", "2nd", "3rd", "4th"})  [unwired: 1 in, 1 out]
              n202 = Greater Or Equal?(x=w691, y=3) -> (x >= y?=w689:bool)
              n203 = Equal?(x=w692, y=w693) -> (x = y?=w699:bool)
              n204 = And(x=w699, y=w694) -> (x .and. y?=w687:bool)
              n205 = Or(x=w687, y=w689) -> (x .or. y?=w688:bool)
              n206 = case shown="True" w687 {
                tunnel: w698 -> [_ w703]
                tunnel: w697 -> [_ w702]
                tunnel: w693 -> [_ w701]
                tunnel: w686 -> [_ w700]
                frame False {
                }
                frame True {
                  n207 = property class="Enum (strict)"(reference=w703, "Value"=w701) -> ()  [unwired: 1 in, 2 out]
                  n208 = property class="Enum (strict)"(reference=w702, "Value"=w700) -> ()  [unwired: 1 in, 2 out]
                }
              }
            }
          }
        }
        n209 = event shown="[1] \"End:Pixel:Order\", \"End:Line:Order\", \"End:Frame:Order\", \"End:Aux:Order\": Value Change" {
          selector: _ -> [_ _]
          dyn-events: _ -> [_ _]
          timeout: 1 -> [_ _]
          tunnel: w620 -> [_ w663]
          event Timeout {
            n210 = event-data() -> ()  [unwired: 3 out]
          }
          event "End:Pixel:Order", "End:Line:Order", "End:Frame:Order", "End:Aux:Order": Value Change {
            n211 = event-data() -> ("CtlRef"=w662:refnum<vi>, "OldVal"=w660:enum16{"1st", "2nd", "3rd", "4th"})  [unwired: 5 out]
            n212 = Unbundle(w663) -> (w661:refnum<vi>[])  [unwired: 3 out]
            n213 = Delete From Array(array=w661, length=4, index=0) -> (array with subset deleted=w659:refnum<vi>[])  [unwired: 1 out]
            n214 = while {
              tunnel: w662 -> [w674]
              tunnel: w659 -> [w673] mode=indexing
              tunnel: w660 -> [w664]
              i -> [w669]
              stop <- w666 stop-if-true
              n215 = Not Equal?(x=w674, y=w673) -> (x != y?=w672:bool)
              n216 = property class="Enum (strict)"(reference=w674) -> (reference out=w676:refnum<vi>, "Value"=w670:enum16{"1st", "2nd", "3rd", "4th"})  [unwired: 1 in, 1 out]
              n217 = property class="Enum (strict)"(reference=w673) -> (reference out=w675:refnum<vi>, "Value"=w671:enum16{"1st", "2nd", "3rd", "4th"})  [unwired: 1 in, 1 out]
              n218 = Greater Or Equal?(x=w669, y=3) -> (x >= y?=w667:bool)
              n219 = Equal?(x=w670, y=w671) -> (x = y?=w677:bool)
              n220 = And(x=w677, y=w672) -> (x .and. y?=w665:bool)
              n221 = Or(x=w665, y=w667) -> (x .or. y?=w666:bool)
              n222 = case shown="True" w665 {
                tunnel: w676 -> [_ w681]
                tunnel: w675 -> [_ w680]
                tunnel: w671 -> [_ w679]
                tunnel: w664 -> [_ w678]
                frame False {
                }
                frame True {
                  n223 = property class="Enum (strict)"(reference=w681, "Value"=w679) -> ()  [unwired: 1 in, 2 out]
                  n224 = property class="Enum (strict)"(reference=w680, "Value"=w678) -> ()  [unwired: 1 in, 2 out]
                }
              }
            }
          }
        }
      }
      frame True {
        n225 = property on="View Start of Scan ISS Commands" class="Bool (strict)"("Visible"=TRUE) -> ()  [unwired: 2 in, 2 out]
        n226 = Compound Arithmetic op=ADD("ISS msStart 1", "ISS msStart 2", "ISS msStart 3", "ISS msStart 4", "ISS msStart 5", "ISS msStart 6", "ISS msStart 7", "ISS msStart 8", "ISS msStart 9", "ISS msStart 10", "ISS msStart 11") -> (→"ISSAdv Start":dbl)
        n227 = control-ref of="PixStartAdv 1"() -> (w736:refnum<vi>)
        n228 = control-ref of="PixStartAdv 2"() -> (w737:refnum<vi>)
        n229 = control-ref of="PixStartAdv 3"() -> (w738:refnum<vi>)
        n230 = control-ref of="PixStartAdv 4"() -> (w739:refnum<vi>)
        n231 = control-ref of="PixStartAdv 5"() -> (w740:refnum<vi>)
        n232 = control-ref of="PixStartAdv 6"() -> (w741:refnum<vi>)
        n233 = control-ref of="PixStartAdv 7"() -> (w742:refnum<vi>)
        n234 = control-ref of="PixStartAdv 8"() -> (w743:refnum<vi>)
        n235 = control-ref of="PixStartAdv 9"() -> (w744:refnum<vi>)
        n236 = control-ref of="PixStartAdv 10"() -> (w745:refnum<vi>)
        n237 = control-ref of="PixStartAdv 11"() -> (w746:refnum<vi>)
        n238 = control-ref of="ISS msStart 1"() -> (w725:refnum<vi>)
        n239 = control-ref of="ISS msStart 2"() -> (w726:refnum<vi>)
        n240 = control-ref of="ISS msStart 3"() -> (w727:refnum<vi>)
        n241 = control-ref of="ISS msStart 4"() -> (w728:refnum<vi>)
        n242 = control-ref of="ISS msStart 5"() -> (w729:refnum<vi>)
        n243 = control-ref of="ISS msStart 6"() -> (w730:refnum<vi>)
        n244 = control-ref of="ISS msStart 7"() -> (w731:refnum<vi>)
        n245 = control-ref of="ISS msStart 8"() -> (w732:refnum<vi>)
        n246 = control-ref of="ISS msStart 9"() -> (w733:refnum<vi>)
        n247 = control-ref of="ISS msStart 10"() -> (w734:refnum<vi>)
        n248 = control-ref of="ISS msStart 11"() -> (w735:refnum<vi>)
        n249 = Select(t=enum32{"Basic", "Adv. Start", "Adv. End"}."Adv. End", s="View Start of Scan ISS Commands", f=enum32{"Basic", "Adv. Start", "Adv. End"}."Adv. Start" ("ISS pre-post config.")) -> (s? t:f=→"ISS pre-post config.":enum32{"Basic", "Adv. Start", "Adv. End"})
        n250 = Build Array(w725, w726, w727, w728, w729, w730, w731, w732, w733, w734, w735) -> (w780:refnum<vi>[])
        n251 = Build Array(w736, w737, w738, w739, w740, w741, w742, w743, w744, w745, w746) -> (w781:refnum<vi>[])
        n252 = control-ref of="FrameStartAdv 1"() -> (w758:refnum<vi>)
        n253 = control-ref of="FrameStartAdv 2"() -> (w759:refnum<vi>)
        n254 = control-ref of="FrameStartAdv 3"() -> (w760:refnum<vi>)
        n255 = control-ref of="FrameStartAdv 4"() -> (w761:refnum<vi>)
        n256 = control-ref of="FrameStartAdv 5"() -> (w762:refnum<vi>)
        n257 = control-ref of="FrameStartAdv 6"() -> (w763:refnum<vi>)
        n258 = control-ref of="FrameStartAdv 7"() -> (w764:refnum<vi>)
        n259 = control-ref of="FrameStartAdv 8"() -> (w765:refnum<vi>)
        n260 = control-ref of="FrameStartAdv 9"() -> (w766:refnum<vi>)
        n261 = control-ref of="FrameStartAdv 10"() -> (w767:refnum<vi>)
        n262 = control-ref of="FrameStartAdv 11"() -> (w768:refnum<vi>)
        n263 = control-ref of="LineStartAdv 1"() -> (w747:refnum<vi>)
        n264 = control-ref of="LineStartAdv 2"() -> (w748:refnum<vi>)
        n265 = control-ref of="LineStartAdv 3"() -> (w749:refnum<vi>)
        n266 = control-ref of="LineStartAdv 4"() -> (w750:refnum<vi>)
        n267 = control-ref of="LineStartAdv 5"() -> (w751:refnum<vi>)
        n268 = control-ref of="LineStartAdv 6"() -> (w752:refnum<vi>)
        n269 = control-ref of="LineStartAdv 7"() -> (w753:refnum<vi>)
        n270 = control-ref of="LineStartAdv 8"() -> (w754:refnum<vi>)
        n271 = control-ref of="LineStartAdv 9"() -> (w755:refnum<vi>)
        n272 = control-ref of="LineStartAdv 10"() -> (w756:refnum<vi>)
        n273 = control-ref of="LineStartAdv 11"() -> (w757:refnum<vi>)
        n274 = Build Array(w747, w748, w749, w750, w751, w752, w753, w754, w755, w756, w757) -> (w782:refnum<vi>[])
        n275 = Build Array(w758, w759, w760, w761, w762, w763, w764, w765, w766, w767, w768) -> (w783:refnum<vi>[])
        n276 = control-ref of="AuxStartAdv 1"() -> (w769:refnum<vi>)
        n277 = control-ref of="AuxStartAdv 2"() -> (w770:refnum<vi>)
        n278 = control-ref of="AuxStartAdv 3"() -> (w771:refnum<vi>)
        n279 = control-ref of="AuxStartAdv 4"() -> (w772:refnum<vi>)
        n280 = control-ref of="AuxStartAdv 5"() -> (w773:refnum<vi>)
        n281 = control-ref of="AuxStartAdv 6"() -> (w774:refnum<vi>)
        n282 = control-ref of="AuxStartAdv 7"() -> (w775:refnum<vi>)
        n283 = control-ref of="AuxStartAdv 8"() -> (w776:refnum<vi>)
        n284 = control-ref of="AuxStartAdv 9"() -> (w777:refnum<vi>)
        n285 = control-ref of="AuxStartAdv 10"() -> (w778:refnum<vi>)
        n286 = control-ref of="AuxStartAdv 11"() -> (w779:refnum<vi>)
        n287 = Build Array(w769, w770, w771, w772, w773, w774, w775, w776, w777, w778, w779) -> (w784:refnum<vi>[])
        n288 = Bundle(w780, w781, w782, w783, w784) -> (w724:T27)  [unwired: 1 out]
        n289 = control-ref of="PixEndAdv 1"() -> (w801:refnum<vi>)
        n290 = control-ref of="PixEndAdv 2"() -> (w802:refnum<vi>)
        n291 = control-ref of="PixEndAdv 3"() -> (w803:refnum<vi>)
        n292 = control-ref of="PixEndAdv 4"() -> (w804:refnum<vi>)
        n293 = control-ref of="PixEndAdv 5"() -> (w805:refnum<vi>)
        n294 = control-ref of="PixEndAdv 6"() -> (w806:refnum<vi>)
        n295 = control-ref of="PixEndAdv 7"() -> (w807:refnum<vi>)
        n296 = control-ref of="PixEndAdv 8"() -> (w808:refnum<vi>)
        n297 = control-ref of="PixEndAdv 9"() -> (w809:refnum<vi>)
        n298 = control-ref of="PixEndAdv 10"() -> (w810:refnum<vi>)
        n299 = control-ref of="PixEndAdv 11"() -> (w811:refnum<vi>)
        n300 = control-ref of="ISS msEnd 1"() -> (w790:refnum<vi>)
        n301 = control-ref of="ISS msEnd 2"() -> (w791:refnum<vi>)
        n302 = control-ref of="ISS msEnd 3"() -> (w792:refnum<vi>)
        n303 = control-ref of="ISS msEnd 4"() -> (w793:refnum<vi>)
        n304 = control-ref of="ISS msEnd 5"() -> (w794:refnum<vi>)
        n305 = control-ref of="ISS msEnd 6"() -> (w795:refnum<vi>)
        n306 = control-ref of="ISS msEnd 7"() -> (w796:refnum<vi>)
        n307 = control-ref of="ISS msEnd 8"() -> (w797:refnum<vi>)
        n308 = control-ref of="ISS msEnd 9"() -> (w798:refnum<vi>)
        n309 = control-ref of="ISS msEnd 10"() -> (w799:refnum<vi>)
        n310 = control-ref of="ISS msEnd 11"() -> (w800:refnum<vi>)
        n311 = Build Array(w790, w791, w792, w793, w794, w795, w796, w797, w798, w799, w800) -> (w789:refnum<vi>[])
        n312 = Build Array(w801, w802, w803, w804, w805, w806, w807, w808, w809, w810, w811) -> (w788:refnum<vi>[])
        n313 = control-ref of="FrameEndAdv 1"() -> (w823:refnum<vi>)
        n314 = control-ref of="FrameEndAdv 2"() -> (w824:refnum<vi>)
        n315 = control-ref of="FrameEndAdv 3"() -> (w825:refnum<vi>)
        n316 = control-ref of="FrameEndAdv 4"() -> (w826:refnum<vi>)
        n317 = control-ref of="FrameEndAdv 5"() -> (w827:refnum<vi>)
        n318 = control-ref of="FrameEndAdv 6"() -> (w828:refnum<vi>)
        n319 = control-ref of="FrameEndAdv 7"() -> (w829:refnum<vi>)
        n320 = control-ref of="FrameEndAdv 8"() -> (w830:refnum<vi>)
        n321 = control-ref of="FrameEndAdv 9"() -> (w831:refnum<vi>)
        n322 = control-ref of="FrameEndAdv 10"() -> (w832:refnum<vi>)
        n323 = control-ref of="FrameEndAdv 11"() -> (w833:refnum<vi>)
        n324 = control-ref of="LineEndAdv 1"() -> (w812:refnum<vi>)
        n325 = control-ref of="LineEndAdv 2"() -> (w813:refnum<vi>)
        n326 = control-ref of="LineEndAdv 3"() -> (w814:refnum<vi>)
        n327 = control-ref of="LineEndAdv 4"() -> (w815:refnum<vi>)
        n328 = control-ref of="LineEndAdv 5"() -> (w816:refnum<vi>)
        n329 = control-ref of="LineEndAdv 6"() -> (w817:refnum<vi>)
        n330 = control-ref of="LineEndAdv 7"() -> (w818:refnum<vi>)
        n331 = control-ref of="LineEndAdv 8"() -> (w819:refnum<vi>)
        n332 = control-ref of="LineEndAdv 9"() -> (w820:refnum<vi>)
        n333 = control-ref of="LineEndAdv 10"() -> (w821:refnum<vi>)
        n334 = control-ref of="LineEndAdv 11"() -> (w822:refnum<vi>)
        n335 = Build Array(w812, w813, w814, w815, w816, w817, w818, w819, w820, w821, w822) -> (w787:refnum<vi>[])
        n336 = Build Array(w823, w824, w825, w826, w827, w828, w829, w830, w831, w832, w833) -> (w786:refnum<vi>[])
        n337 = control-ref of="AuxEndAdv 1"() -> (w834:refnum<vi>)
        n338 = control-ref of="AuxEndAdv 2"() -> (w835:refnum<vi>)
        n339 = control-ref of="AuxEndAdv 3"() -> (w836:refnum<vi>)
        n340 = control-ref of="AuxEndAdv 4"() -> (w837:refnum<vi>)
        n341 = control-ref of="AuxEndAdv 5"() -> (w838:refnum<vi>)
        n342 = control-ref of="AuxEndAdv 6"() -> (w839:refnum<vi>)
        n343 = control-ref of="AuxEndAdv 7"() -> (w840:refnum<vi>)
        n344 = control-ref of="AuxEndAdv 8"() -> (w841:refnum<vi>)
        n345 = control-ref of="AuxEndAdv 9"() -> (w842:refnum<vi>)
        n346 = control-ref of="AuxEndAdv 10"() -> (w843:refnum<vi>)
        n347 = control-ref of="AuxEndAdv 11"() -> (w844:refnum<vi>)
        n348 = Build Array(w834, w835, w836, w837, w838, w839, w840, w841, w842, w843, w844) -> (w785:refnum<vi>[])
        n349 = Bundle(w789, w788, w787, w786, w785) -> (w723:T27)  [unwired: 1 out]
        n350 = Bundle(w723, w724) -> (w722:T17)  [unwired: 1 out]
      }
    }
    n351 = Not Equal?(x=w172, y="Template") -> (x != y?=w180:bool)
    n352 = Or(x=w170, y=w180) -> (x .or. y?=w171:bool)
    n353 = Bundle("Template"=w172, "Template"="Template", "pulse template"=FALSE) -> (w345:T28)  [unwired: 1 out]
    n354 = for {
      N: 1 -> [_]
      shift-right: [w849] -> _
      shift-left: _ -> [w848]
      tunnel: [w845] -> w190
      n355 = Increment(x=w848) -> (x+1=w847:i32)
      n356 = Equal?(x=10, y=w848) -> (x = y?=w845:bool)
      n357 = Select(t=0, s=w845, f=w847) -> (s? t:f=w849:i32)
    }
    n358 = case shown="True" w171 {
      tunnel: w316 -> [_ w514]
      tunnel: "Template" -> [_ w512]
      frame False {
      }
      frame True {
        n359 = case shown="1" w512 {
          tunnel: [w529 w540 w548 u8 2 ("Disabled") u8 0 ("Disabled") u8 0 ("Disabled") u8 0 ("Disabled")] -> w524
          tunnel: [w528 u8 2 ("A/D Rate\n16-bit") u8 2 ("A/D Rate\n16-bit") w553 u8 0 ("A/D Rate\n16-bit") u8 0 ("A/D Rate\n16-bit") u8 0 ("A/D Rate\n16-bit")] -> w523
          tunnel: [u8 0 ("A/D Rate\n16-bit") u8 0 ("A/D Rate\n16-bit") w547 w554 u8 0 ("A/D Rate\n16-bit") u8 0 ("A/D Rate\n16-bit") u8 0 ("A/D Rate\n16-bit")] -> w522
          tunnel: [u8 0 ("Disabled") u8 2 ("Disabled") w548 w556 w567 w577 w587] -> w521
          tunnel: [w529 w540 w548 u8 0 ("A/D Rate\n16-bit") u8 0 ("A/D Rate\n16-bit") u8 0 ("A/D Rate\n16-bit") u8 0 ("A/D Rate\n16-bit")] -> w520
          tunnel: [u8 0 ("A/D Rate\n16-bit") u8 2 ("A/D Rate\n16-bit") w547 u8 0 ("A/D Rate\n16-bit") u8 0 ("A/D Rate\n16-bit") u8 0 ("A/D Rate\n16-bit") u8 0 ("A/D Rate\n16-bit")] -> w519
          tunnel: [w529 u8 0 ("Disabled") w548 w556 w567 w577 w587] -> w518
          tunnel: [w528 u8 0 ("A/D Rate\n16-bit") u8 0 ("A/D Rate\n16-bit") w554 u8 0 ("A/D Rate\n16-bit") u8 0 ("A/D Rate\n16-bit") u8 0 ("A/D Rate\n16-bit")] -> w517
          tunnel: [u8 2 ("A/D Rate\n16-bit") u8 2 ("A/D Rate\n16-bit") u8 2 ("A/D Rate\n16-bit") w553 u8 2 ("A/D Rate\n16-bit") u8 2 ("A/D Rate\n16-bit") u8 2 ("A/D Rate\n16-bit")] -> w516
          tunnel: [FALSE ("Visible") FALSE ("Visible") FALSE ("Visible") TRUE ("Visible") FALSE ("Visible") FALSE ("Visible") FALSE ("Visible")] -> w515
          tunnel: w514 -> [_ _ _ _ _ _ _]
          tunnel: [T3."Raster Scan" ("Custom Scans") T3."Empty" ("Custom Scans") T3."Empty" ("Custom Scans") T3."Raster Scan" ("Custom Scans") T3."Raster Scan" ("Custom Scans") T3."Custom 1" ("Custom Scans") T3."Custom 2" ("Custom Scans")] -> w513
          frame 0, Default {
            w528 = u8 0 ("A/D Rate\n16-bit")
            w529 = u8 0 ("Disabled")
          }
          frame 1 {
            w540 = u8 0 ("Disabled")
          }
          frame 2 {
            w547 = u8 2 ("A/D Rate\n16-bit")
            w548 = u8 0 ("Disabled")
            n360 = local write "WF\nAcq."(FALSE ("WF\nAcq.")) -> ()
          }
          frame 3 {
            w555 = u8 1 items=["ms", "dpts"] ("Path Units")
            w554 = u8 2 ("A/D Rate\n16-bit")
            w556 = u8 2 ("Disabled")
            w553 = u8 0 ("A/D Rate\n16-bit")
            w561 = 1.0 ("A/D Rate\n16-bit")
            n361 = local write "A/D Rate\n16-bit"(w561) -> ()
            n362 = local write "A/D Rate\n20-bit"(w561) -> ()
            n363 = local write "WF\nAcq."(FALSE ("WF\nAcq.")) -> ()
            n364 = local write "Path Units"(w555) -> ()
          }
          frame 4 {
            w567 = u8 0 ("Disabled")
          }
          frame 5 {
            w577 = u8 0 ("Disabled")
          }
          frame 6 {
            w587 = u8 0 ("Disabled")
          }
        }
        n365 = stacked-sequence {
          tunnel: w524 -> [w593 _ _ _ _ _ _]
          tunnel: w523 -> [_ _ _ w604 w610 _ _]
          tunnel: w522 -> [_ _ w601 _ _ _ _]
          tunnel: w521 -> [_ w598 _ _ _ _ _]
          tunnel: w520 -> [_ _ w602 _ _ _ _]
          tunnel: w519 -> [_ _ _ w606 _ _ _]
          tunnel: w518 -> [_ w596 _ _ _ _ _]
          tunnel: w517 -> [_ w595 _ _ _ _ _]
          tunnel: w516 -> [_ _ _ _ _ w612 _]
          tunnel: w515 -> [_ _ _ _ _ w611 _]
          tunnel: w513 -> [w592 _ _ _ _ _ _]
          frame #0 {
            n366 = property on="A/D Rate\n16-bit" class="DigNum (strict)"("Disabled"=w593) -> ()  [unwired: 2 in, 2 out]
            n367 = property on="A/D Rate\n20-bit" class="Ring (strict)"("Disabled"=w593) -> ()  [unwired: 2 in, 2 out]
            "Custom Scans" <- w592
          }
          frame #1 {
            n368 = property on="Path Units" class="Ring (strict)"("Disabled"=w595) -> ()  [unwired: 2 in, 2 out]
            n369 = property on="Run All Routes" class="Bool"("Disabled"=w598) -> ()  [unwired: 2 in, 2 out]
            n370 = property on="Run Route" class="Bool"("Disabled"=w596) -> ()  [unwired: 2 in, 2 out]
            n371 = Equal To 0?(x=w595) -> (x = 0?=w594:bool)
            n372 = Equal To 0?(x=w598) -> (x = 0?=w599:bool)
            n373 = Equal To 0?(x=w596) -> (x = 0?=w597:bool)
            n374 = property on="Run All Routes" class="Bool"("Visible"=w599) -> ()  [unwired: 2 in, 2 out]
            n375 = property on="Path Units" class="Ring (strict)"("Visible"=w594) -> ()  [unwired: 2 in, 2 out]
            n376 = property on="Run Route" class="Bool"("Visible"=w597) -> ()  [unwired: 2 in, 2 out]
          }
          frame #2 {
            n377 = property on="AddPath" class="Bool"("Disabled"=w602) -> ()  [unwired: 2 in, 2 out]
            n378 = property on="DeletePath" class="Bool"("Disabled"=w602) -> ()  [unwired: 2 in, 2 out]
            n379 = property on="Load Route" class="Bool"("Disabled"=w602) -> ()  [unwired: 2 in, 2 out]
            n380 = property on="Reset" class="Bool"("Disabled"=w602) -> ()  [unwired: 2 in, 2 out]
            n381 = property on="WF\nAcq." class="Bool (strict)"("Disabled"=w601) -> ()  [unwired: 2 in, 2 out]
            n382 = Equal To 0?(x=w601) -> (x = 0?=w600:bool)
            n383 = Equal To 0?(x=w602) -> ()  [unwired: 1 out]
            n384 = property on="WF\nAcq." class="Bool (strict)"("Visible"=w600) -> ()  [unwired: 2 in, 2 out]
          }
          frame #3 {
            n385 = property on="Pixel delay" class="DigNum (strict)"("Disabled"=w604) -> ()  [unwired: 2 in, 2 out]
            n386 = property on="Pixel" class="Ring (strict)"("Disabled"=w604) -> ()  [unwired: 2 in, 2 out]
            n387 = property on="Line" class="Ring (strict)"("Disabled"=w604) -> ()  [unwired: 2 in, 2 out]
            n388 = property on="Frame" class="Ring (strict)"("Disabled"=w604) -> ()  [unwired: 2 in, 2 out]
            n389 = property on="Begin Raster" class="Bool (strict)"("Disabled"=w606) -> ()  [unwired: 2 in, 2 out]
            n390 = Equal To 0?(x=w606) -> (x = 0?=w605:bool)
            n391 = Equal To 0?(x=w604) -> (x = 0?=w603:bool)
            n392 = property on="Begin Raster" class="Bool (strict)"("Visible"=w605) -> ()  [unwired: 2 in, 2 out]
            n393 = property on="Pixel delay" class="DigNum (strict)"("Visible"=w603) -> ()  [unwired: 2 in, 2 out]
            n394 = property on="Pixel" class="Ring (strict)"("Visible"=w603) -> ()  [unwired: 2 in, 2 out]
            n395 = property on="Line" class="Ring (strict)"("Visible"=w603) -> ()  [unwired: 2 in, 2 out]
            n396 = property on="Frame" class="Ring (strict)"("Visible"=w603) -> ()  [unwired: 2 in, 2 out]
          }
          frame #4 {
            n397 = property on="End of Line delay" class="DigNum (strict)"("Disabled"=w610) -> ()  [unwired: 2 in, 2 out]
            n398 = property on="Start of Line delay" class="DigNum (strict)"("Disabled"=w610) -> ()  [unwired: 2 in, 2 out]
            n399 = property on="Frame delay" class="DigNum (strict)"("Disabled"=w610) -> ()  [unwired: 2 in, 2 out]
            n400 = property on="Est. R.S. time" class="DigNum (strict)"("Disabled"=w610) -> ()  [unwired: 2 in, 2 out]
            n401 = property on="Mirror motion on return?" class="Bool (strict)"("Disabled"=w610) -> ()  [unwired: 2 in, 2 out]
            n402 = Equal To 0?(x=w610) -> (x = 0?=w609:bool)
            n403 = property on="End of Line delay" class="DigNum (strict)"("Visible"=w609) -> ()  [unwired: 2 in, 2 out]
            n404 = property on="Start of Line delay" class="DigNum (strict)"("Visible"=w609) -> ()  [unwired: 2 in, 2 out]
            n405 = property on="Frame delay" class="DigNum (strict)"("Visible"=w609) -> ()  [unwired: 2 in, 2 out]
            n406 = property on="Mirror motion on return?" class="Bool (strict)"("Visible"=w609) -> ()  [unwired: 2 in, 2 out]
            n407 = property on="Est. R.S. time" class="DigNum (strict)"("Visible"=w609) -> ()  [unwired: 2 in, 2 out]
            n408 = Select(t="Raster Scan" ("Custom.name"), s=w609, f="") -> ()  [unwired: 1 out]
          }
          frame #5 {
            n409 = property on="Ignore" class="Bool"("Disabled"=w612) -> ()  [unwired: 2 in, 2 out]
            n410 = property on="Ignore" class="Bool"("Visible"=w611) -> ()  [unwired: 2 in, 2 out]
          }
          frame #6 {
          }
        }
      }
    }
    n411 = control-ref of="X Calibration 2"() -> (w243:refnum<vi>)
    n412 = control-ref of="Y Calibration 2"() -> (w242:refnum<vi>)
    n413 = control-ref of="Z Calibration 2"() -> (w241:refnum<vi>)
    n414 = control-ref of="Aux Calibration 2"() -> (w240:refnum<vi>)
    n415 = control-ref of="Dll Revision"() -> (w239:refnum<vi>)
    n416 = control-ref of="ADC Freq (ms)"() -> (w238:refnum<vi>)
    n417 = control-ref of="DAC Freq (ms)"() -> (w237:refnum<vi>)
    n418 = control-ref of="Serial # 2"() -> (w236:refnum<vi>)
    n419 = stacked-sequence {
      tunnel: w370 -> [_ _]
      frame #0 {
        # "Flashing Red Plot"
        n420 = property on="Route Graph" class="XYGraph (strict)"("Active Plot"=u32 1) -> ()  [unwired: 2 in, 2 out]
      }
      frame #1 {
        # "Flashing Red Plot"
        n421 = call "_nr_AltBool.vi"("1 = fast\n10 = slow"=u16 3 ("y")) -> ("Alternating\nBoolean"=w1474:bool)
        n422 = property on="Route Graph" class="XYGraph (strict)"("Plot.Visible?"=w1474) -> ()  [unwired: 2 in, 2 out]
      }
    }
    n423 = To Long Integer(number="Axis") -> (32bit integer=w111:i32)
    n424 = Unbundle(w80) -> ("Incoming Handle"=w153:i32)  [unwired: 2 out]
    n425 = Decrement(x=w111) -> (x-1=w112:i32)
    n426 = case shown="True" "LivePosition" {
      tunnel: w334 -> [_ w856]
      tunnel: w146 -> [_ w855]
      tunnel: w78 -> [_ w854]
      tunnel: [enum32{"disable", "enable"}."disable" ("LivePosition") enum32{"disable", "enable"}."enable" ("LivePosition")] -> w199
      tunnel: w190 -> [_ w852]
      frame False {
      }
      frame True {
        n427 = case shown="True" w852 {
          tunnel: w854 -> [_ w865]
          tunnel: w856 -> [_ w864]
          tunnel: w855 -> [_ w857]
          frame False {
          }
          frame True {
            n428 = call "_nr_ConstantRead.vi"("Command X"="Command X", "X command"="X command", "ISS Info"=w857, "Command Y"="Command Y", "Y command"="Y command", "Command Z"="Command Z", "handle"=w864, "Z command"="Z command", "Active Axes"=w865) -> ("X-Axis"=→"X-Axis":dbl, "Y-Axis"=→"Y-Axis":dbl, "Z-Axis"=→"Z-Axis":dbl)  [unwired: 4 out]
          }
        }
      }
    }
    "LivePosition" <- w199
    n429 = Build Array(w112) -> (w113:i32[])
    n430 = case shown="True" "gamepad" {
      tunnel: w153 -> [_ w453]
      tunnel: w146 -> [_ w454]
      frame False {
      }
      frame True {
        n431 = flat-sequence {
          tunnel: [w461] -> w458
          tunnel: [w460] -> w457
          tunnel: w453 -> [w459]
          tunnel: w454 -> [w460]
          tunnel: w458 -> [w483]
          tunnel: w457 -> [w484]
          tunnel: [w483] -> w456
          tunnel: [w484] -> w455
          tunnel: w456 -> [w486]
          tunnel: w455 -> [w485]
          frame #0 {
            n432 = Unbundle(w460) -> ("ISS Confirmed Options"=w469:T29, "ISS Confirmed Options"=w468:T29, "ISS Confirmed Options"=w467:T29, "ISS Confirmed Options"=w466:T29)  [unwired: 1 out]
            n433 = Unbundle By Name(w467) -> ("Pixel Polarity"=w464:enum16{"Low", "High"})
            n434 = Unbundle By Name(w469) -> ("Pixel Polarity"=w462:enum16{"Low", "High"})
            n435 = Unbundle By Name(w468) -> ("Pixel Polarity"=w463:enum16{"Low", "High"})
            n436 = Unbundle By Name(w466) -> ("Pixel Polarity"=w465:enum16{"Low", "High"})
            n437 = flat-sequence {
              tunnel: [w472] -> w461
              tunnel: w459 -> [w470]
              tunnel: w465 -> [w471]
              tunnel: w464 -> [w477]
              tunnel: w463 -> [w479]
              tunnel: w462 -> [w481]
              frame #0 {
                n438 = dll-call lib="C:/Users/Labview/Desktop/64-bit VIs/Madlib.dll" fn="MCL_IssSetClock"("clock"=4, "mode"=w471, "handle"=w470) -> ("handle"=w475:i32)  [unwired: 4 in, 4 out]
                n439 = dll-call lib="C:/Users/Labview/Desktop/64-bit VIs/Madlib.dll" fn="MCL_IssSetClock"("clock"=3, "mode"=w477, "handle"=w475) -> ("handle"=w474:i32)  [unwired: 4 in, 4 out]
                n440 = dll-call lib="C:/Users/Labview/Desktop/64-bit VIs/Madlib.dll" fn="MCL_IssSetClock"("clock"=2, "mode"=w479, "handle"=w474) -> ("handle"=w473:i32)  [unwired: 4 in, 4 out]
                n441 = dll-call lib="C:/Users/Labview/Desktop/64-bit VIs/Madlib.dll" fn="MCL_IssSetClock"("clock"=1, "mode"=w481, "handle"=w473) -> ("handle"=w472:i32)  [unwired: 4 in, 4 out]
              }
            }
          }
          frame #1 {
            n442 = call "Gamepad NanoDrive Control.vi"("handle"=w483) -> ()  [unwired: 1 in]
          }
          frame #2 {
            n443 = Unbundle(w485) -> ("ISS Confirmed Options"=w491:T29, "ISS Confirmed Options"=w495:T29, "ISS Confirmed Options"=w499:T29, "ISS Confirmed Options"=w503:T29)  [unwired: 1 out]
            n444 = Unbundle(w491) -> ("Pixel Polarity"=w492:enum16{"Low", "High"}, "Pixel Pulse"=w493:enum16{"Low to High", "High to Low"}, "Pixel Bind"=w494:T4)  [unwired: 1 out]
            n445 = Unbundle(w495) -> ("Pixel Polarity"=w496:enum16{"Low", "High"}, "Pixel Pulse"=w497:enum16{"Low to High", "High to Low"}, "Pixel Bind"=w498:T4)  [unwired: 1 out]
            n446 = Unbundle(w499) -> ("Pixel Polarity"=w500:enum16{"Low", "High"}, "Pixel Pulse"=w501:enum16{"Low to High", "High to Low"}, "Pixel Bind"=w502:T4)  [unwired: 1 out]
            n447 = Unbundle(w503) -> ("Pixel Polarity"=w504:enum16{"Low", "High"}, "Pixel Pulse"=w505:enum16{"Low to High", "High to Low"}, "Pixel Bind"=w506:T4)  [unwired: 1 out]
            n448 = call "_nr_ISS.vi"("Polarity"=w500, "clock (1=Pixel)"=3, "Pulse"=w501, "Axis Binding"=w502, "ISS Confirmed Options (Feedback)"=w499, "Confirm"=TRUE, "Incoming Handle"=w486) -> ()  [unwired: 3 in, 6 out]
            n449 = call "_nr_ISS.vi"("Polarity"=w492, "clock (1=Pixel)"=1, "Pulse"=w493, "Axis Binding"=w494, "ISS Confirmed Options (Feedback)"=w491, "Confirm"=TRUE, "Incoming Handle"=w486) -> ()  [unwired: 3 in, 6 out]
            n450 = call "_nr_ISS.vi"("Polarity"=w496, "clock (1=Pixel)"=2, "Pulse"=w497, "Axis Binding"=w498, "ISS Confirmed Options (Feedback)"=w495, "Confirm"=TRUE, "Incoming Handle"=w486) -> ()  [unwired: 3 in, 6 out]
            n451 = call "_nr_ISS.vi"("Polarity"=w504, "clock (1=Pixel)"=4, "Pulse"=w505, "Axis Binding"=w506, "ISS Confirmed Options (Feedback)"=w503, "Confirm"=TRUE, "Incoming Handle"=w486) -> ()  [unwired: 3 in, 6 out]
          }
        }
      }
    }
    n452 = control-ref of="Route Graph"() -> (w254:refnum<vi>)
    n453 = control-ref of="Route Graph"() -> (w290:refnum<vi>)
    n454 = Bundle("ADC resolution (bits)"=w253, "DAC resolution (bits)"=w252, "Product ID (in hex) 2"=w251, "Firmware Version 2"=w250, "Firmware Profile"=w249, "Dll Version"=w248, "X axis"=w247, "Y axis"=w246, "Z axis"=w245, "Aux axis"=w244, "X Calibration 2"=w243, "Y Calibration 2"=w242, "Z Calibration 2"=w241, "Aux Calibration 2"=w240, "Dll Revision"=w239, "ADC Freq (ms)"=w238, "DAC Freq (ms)"=w237, "Serial # 2"=w236) -> (w235:T30)  [unwired: 1 out]
    n455 = control-ref of="handleIndex"() -> (w291:refnum<vi>)
    n456 = control-ref of="Axis"() -> (w292:refnum<vi>)
    n457 = property on="offset" class="Arr (strict)"("Index Values"=w113) -> ()  [unwired: 2 in, 2 out]
    n458 = case shown="True" w329 {
      selector: w329 -> [w1652 w1689]
      tunnel: w412 -> [w1654 w1697]
      tunnel: [w1651 w1701] -> w365
      tunnel: w419 -> [w1659 _]
      tunnel: [w1646 w1695] -> w414
      tunnel: ["" w1684] -> w415
      tunnel: [w1647 w1696] -> w233
      tunnel: [w1661 w1682] -> w77
      tunnel: w74 -> [_ w1700]
      tunnel: w323 -> [_ w1701]
      tunnel: [w1649 w1685] -> w82
      tunnel: [w1645 w1694] -> w411
      tunnel: [w1643 w1693] -> w410
      tunnel: [w1644 w1683] -> w79
      tunnel: [w1648 w1691] -> w275
      tunnel: [w1662 w1692] -> w324
      tunnel: w322 -> [w1642 w1688]
      tunnel: "handleIndex" -> [w1656 w1699]
      tunnel: w292 -> [w1657 _]
      tunnel: w291 -> [w1658 _]
      tunnel: w290 -> [w1653 w1690]
      tunnel: "Axis" -> [w1655 w1698]
      tunnel: w254 -> [w1660 _]
      tunnel: w235 -> [w1640 w1666]
      frame False {
        n459 = Unbundle(w1642) -> ("handleIndex"=w1641:i32)  [unwired: 2 out]
        n460 = call "_nr_DeviceInfoSubvi.vi"(0:"handleIndex"=w1656, "previous handleIndex"=w1641, 3:"Axis"=w1655, "Cluster 2"=w1642, "Incoming Handle"=w1654, "Build Graph"=w1653, "x .and. y?"=w1659, "Device Loaded?"=w1652, "Route Graph 2"=w1660, 15:"handleIndex"=w1658, 17:"Axis"=w1657) -> ("Device Loaded"=w1651:bool, "Device Info"=w1650:T31, "Outgoing Handle"=w1661:i32, "Handles List"=w1662:T32)  [unwired: 1 in, 12 out]
        n461 = call "_nr_DeviceInfoDisplay.vi"("Device Info Control References"=w1640, "Device Info IN"=w1650) -> ("Device Info OUT"=w1649:T31, "20 bit"=w1648:bool, "Serial #"=w1647:string, "Existing Axes"=w1644:T6, "X Calibration"=w1646:dbl, "Z Calibration"=w1643:dbl, "Y Calibration"=w1645:dbl)  [unwired: 7 out]
      }
      frame True {
        n462 = Unbundle(w1688) -> ("handleIndex"=w1687:i32)  [unwired: 2 out]
        n463 = call "_nr_DeviceInfoSubvi.vi"("handleIndex"=w1699, "previous handleIndex"=w1687, "Axis"=w1698, "Cluster 2"=w1688, "Incoming Handle"=w1697, "Build Graph"=w1690, "Cluster"=w1700, "Device Loaded?"=w1689) -> ("20bit"=w1691:bool, "Device Info"=w1686:T31, "Text"=w1696:string, "X Calibration"=w1695:dbl, "Y Calibration"=w1694:dbl, "Z Calibration"=w1693:dbl, "Outgoing Handle"=w1682:i32, "Handles List"=w1692:T32)  [unwired: 4 in, 8 out]
        n464 = control-ref of="include 1"() -> (w1668:refnum<vi>)
        n465 = control-ref of="include 2"() -> (w1669:refnum<vi>)
        n466 = control-ref of="include 3"() -> (w1670:refnum<vi>)
        n467 = control-ref of="include 4"() -> (w1671:refnum<vi>)
        n468 = control-ref of="include 5"() -> (w1672:refnum<vi>)
        n469 = control-ref of="include 6"() -> (w1673:refnum<vi>)
        n470 = control-ref of="include 7"() -> (w1674:refnum<vi>)
        n471 = control-ref of="include 8"() -> (w1675:refnum<vi>)
        n472 = control-ref of="include 9"() -> (w1676:refnum<vi>)
        n473 = control-ref of="include 10"() -> (w1677:refnum<vi>)
        n474 = control-ref of="include 11"() -> (w1678:refnum<vi>)
        n475 = control-ref of="include 12"() -> (w1679:refnum<vi>)
        n476 = control-ref of="include 13"() -> (w1680:refnum<vi>)
        n477 = control-ref of="include 14"() -> (w1681:refnum<vi>)
        n478 = Bundle("include 1"=w1668, "include 2"=w1669, "include 3"=w1670, "include 4"=w1671, "include 5"=w1672, "include 6"=w1673, "include 7"=w1674, "include 8"=w1675, "include 9"=w1676, "include 10"=w1677, "include 11"=w1678, "include 12"=w1679, "include 13"=w1680, "include 14"=w1681) -> (w1667:T33)  [unwired: 1 out]
        n479 = call "_nr_DeviceInfoDisplay2.vi"("Device Info Control References"=w1666, "Include Button References"=w1667, "Handle"=w1682, "Remove All 2"="Set All", "Set All 2"="Remove All", "Device Info IN"=w1686) -> ("Active Axes"=w1683:T6, "Concatenated Device Info String"=w1684:string, "Device Info OUT"=w1685:T31)  [unwired: 3 out]
      }
    }
    "Device Data" <- w415
    n480 = local read "offset"() -> (w115:dbl[])
    n481 = local read "Axis"() -> (w116:u32)
    n482 = case shown="True" w317 {
      tunnel: w178 -> [w1220 w1224]
      tunnel: [w1220 w1225] -> w224
      tunnel: w231 -> [_ w1223]
      tunnel: [FALSE ("Pixel uses Waveform Acquisition OUT") w1221] -> w182
      frame False {
      }
      frame True {
        n483 = call "_nrDialog_RasterScanAdvConf.vi"("Enable"=TRUE, "20bit"=w1223, "Raster Scan Advanced Options IN"=w1224) -> ("Pixel uses Waveform Acquisition OUT"=w1221:bool, "Raster Scan Advanced Options OUT"=w1225:T8)  [unwired: 15 out]
      }
    }
    n484 = Bundle("Mirror motion on return?"=w223, "Raster Scan Advanced Options OUT"=w224, "RasterAxisConfig"=w69, "RasterDelays"=w68) -> (w222:T34)  [unwired: 1 out]
    n485 = Bundle("Pixel delay"=w383, "End of Line delay"=w382, "Start of Line delay"=w380, "Frame delay"=w381, "Pixel dwell"=w142) -> (w70:T5)  [unwired: 1 out]
    n486 = Decrement(x=w116) -> (x-1=w117:u32)
    n487 = local read "Relative Start"() -> (w157:bool)
    n488 = Index Array(array=w115, index=w117) -> (element=w114:dbl)
    n489 = call "_nr_GeneratePath.vi"("Path Parameters"=w396) -> ("function array"=w264:cluster{dbl[], dbl[]})  [unwired: 1 in, 1 out]
    n490 = Unbundle(w74) -> ("20bit"=w262:bool)  [unwired: 5 out]
    n491 = case shown="True" w262 {
      tunnel: w76 -> [_ w1591]
      tunnel: w179 -> [_ w1589]
      frame False {
      }
      frame True {
        n492 = dll-call lib="C:/Users/Labview/Desktop/64-bit VIs/Madlib.dll" fn="MCL_ChangeClock"("milliseconds"=w1589, "True = DAC"=i8 0, "handle"=w1591) -> ()  [unwired: 6 in, 3 out]
      }
    }
    n493 = case shown="True" w182 {
      frame False {
      }
      frame True {
        n494 = property on="Path Units" class="Ring (strict)"("Value"=u8 1 ("Disabled")) -> ()  [unwired: 2 in, 2 out]
      }
    }
    n495 = Bundle("Relative Start"=w157, "offset"=w114, "Incoming Handle"=w156) -> (w155:T35)  [unwired: 1 out]
    n496 = case shown="3" w266 {
      tunnel: string[] ["Point by Point", "Time in milliseconds", "Axis: X Position", "Axis: Y Position", "Axis: Z Position"] ("Strings []") -> [w1595 w1597 _ w1603]
      tunnel: [w1595 w1597 w1600 w1603] -> w385
      tunnel: [w1595 w1597 w1600 w1603] -> w384
      tunnel: string[] ["Point by Point", "Time in milliseconds", "Frame", "Line", "Pixel"] ("Strings []") -> [_ _ w1600 _]
      tunnel: [u8 0 ("Disabled") u8 0 ("Disabled") u8 2 ("Disabled") u8 0 ("Disabled")] -> w162
      frame 0, Default {
        n497 = property on="X-Axis Display" class="Ring (strict)"("Disabled Items []"=i32[] [2, 3, 4]) -> ()  [unwired: 2 in, 2 out]
        n498 = property on="Y-Axis Display" class="Ring (strict)"("Disabled Items []"=i32[] [0, 1]) -> ()  [unwired: 2 in, 2 out]
      }
      frame 1 {
        w1598 = i32[] [] ("Disabled Items []")
        n499 = property on="X-Axis Display" class="Ring (strict)"("Disabled Items []"=w1598) -> ()  [unwired: 2 in, 2 out]
        n500 = property on="Y-Axis Display" class="Ring (strict)"("Disabled Items []"=w1598) -> ()  [unwired: 2 in, 2 out]
      }
      frame 2 {
        w1601 = i32[] [] ("Disabled Items []")
        n501 = property on="X-Axis Display" class="Ring (strict)"("Disabled Items []"=w1601) -> ()  [unwired: 2 in, 2 out]
        n502 = property on="Y-Axis Display" class="Ring (strict)"("Disabled Items []"=w1601) -> ()  [unwired: 2 in, 2 out]
      }
      frame 3 {
        w1604 = i32[] [] ("Disabled Items []")
        n503 = property on="X-Axis Display" class="Ring (strict)"("Disabled Items []"=w1604) -> ()  [unwired: 2 in, 2 out]
        n504 = property on="Y-Axis Display" class="Ring (strict)"("Disabled Items []"=w1604) -> ()  [unwired: 2 in, 2 out]
      }
    }
    n505 = call "_nr_PrepareRasterdData.vi"("Line"=w287, "Pixel"=w288, "Raster Scan Advanced Options IN"=w224, "Frame"=w286, "20 bit"=w231, "Cluster of Routes"=w300, "Raster delays"=w70, "Begin Raster - unblock RR reading"=w141, "RelativeRoute"=w155) -> ("Pixel Route"=w314:dbl[], "Line Route"=w313:dbl[], "Frame Route"=w312:dbl[], "Estimated\nRaster\nTime"=w307:dbl, "WaveAcq Setup"=w310:T36)  [unwired: 2 in]
    n506 = property on="X-Axis Display" class="Ring (strict)"("Strings []"=w385) -> ()  [unwired: 2 in, 2 out]
    n507 = property on="Y-Axis Display" class="Ring (strict)"("Strings []"=w384) -> ()  [unwired: 2 in, 2 out]
    n508 = Bundle("Pixel"=w288, "Line"=w287, "Frame"=w286) -> (w71:cluster{"Pixel":u32, "Line":u32, "Frame":u32})  [unwired: 1 out]
    n509 = Bundle("Text"=w233, "Device Info OUT"=w82, "X Calibration"=w414, "Y Calibration"=w411, "Z Calibration"=w410, "20bit"=w275) -> (w75:T37)  [unwired: 1 out]
    n510 = property on="Export DAC" class="Bool"("Disabled"=w162) -> ()  [unwired: 2 in, 2 out]
    n511 = flat-sequence {
      tunnel: w397 -> [w1041]
      tunnel: w395 -> [w1040]
      tunnel: w72 -> [w1036]
      tunnel: w280 -> [w1035]
      tunnel: w90 -> [w1034]
      tunnel: w234 -> [w1033]
      tunnel: w179 -> [w1024]
      tunnel: w84 -> [w1032]
      tunnel: w265 -> [w1029]
      tunnel: w264 -> [w1028]
      tunnel: w263 -> [w1025]
      tunnel: [w1043] -> w128
      tunnel: [w1027] -> w126
      tunnel: [w1026] -> w125
      tunnel: [w1025] -> w122
      tunnel: [w1024] -> w119
      tunnel: w128 -> [w1060]
      tunnel: w126 -> [w1059]
      tunnel: w125 -> [w1058]
      tunnel: [w1059] -> w124
      tunnel: [w1058] -> w123
      tunnel: w122 -> [w1057]
      tunnel: [w1057] -> w121
      tunnel: [w1056] -> w120
      tunnel: w119 -> [w1056]
      tunnel: w124 -> [w1063]
      tunnel: w123 -> [w1061]
      tunnel: w121 -> [w1069]
      tunnel: w120 -> [w1065]
      frame #0 {
        # "DISPLAY PATH/ROUTE DATA"
        # "Current Point Highlight"
        # "Route Plot for Current Point"
        n512 = Build Array(w1041) -> (w1045:dbl[])
        n513 = Build Array(w1040) -> (w1044:dbl[])
        n514 = Unbundle(w1028) -> (w1042:dbl[])  [unwired: 1 out]
        n515 = Unbundle(w1029) -> (w1038:dbl[])  [unwired: 1 out]
        n516 = case shown="3" w1036 {
          tunnel: w1032 -> [w1051 w1053 w1055]
          tunnel: [w1050 w1052 w1054] -> w1037
          frame 1, Default {
            n517 = Unbundle(w1051) -> (w1050:cluster{dbl[], dbl[]})  [unwired: 2 out]
          }
          frame 2 {
            n518 = Unbundle(w1053) -> (w1052:cluster{dbl[], dbl[]})  [unwired: 2 out]
          }
          frame 3 {
            n519 = Unbundle(w1055) -> (w1054:cluster{dbl[], dbl[]})  [unwired: 2 out]
          }
        }
        n520 = Array Size(array=w1042) -> (size(s)=w1027:i32)
        "Points in Current Path" <- w1027
        n521 = Array Size(array=w1038) -> (size(s)=w1026:i32)
        "Points in Route" <- w1026
        n522 = case shown="1" w1025 {
          tunnel: w1024 -> [w1047 _]
          tunnel: "Time in Milliseconds" ("X Scale.Name Label.Text") -> [w1046 _]
          tunnel: "Data Point Count" ("X Scale.Name Label.Text") -> [_ w1048]
          frame 0, Default {
            n523 = property on="Route Graph" class="XYGraph (strict)"("XScale.NameLbl.Text"=w1046) -> ()  [unwired: 2 in, 2 out]
            n524 = property on="Route Graph" class="XYGraph (strict)"("XScale.Multiplier"=w1047) -> ()  [unwired: 2 in, 2 out]
          }
          frame 1 {
            n525 = property on="Route Graph" class="XYGraph (strict)"("XScale.NameLbl.Text"=w1048) -> ()  [unwired: 2 in, 2 out]
            n526 = property on="Route Graph" class="XYGraph (strict)"("XScale.Multiplier"=1.0 ("X Scale.Offset and Multiplier:Multiplier")) -> ()  [unwired: 2 in, 2 out]
          }
        }
        n527 = Bundle(w1045, w1044) -> (w1039:cluster{dbl[], dbl[]})  [unwired: 1 out]
        n528 = Build Array(w1039, w1028, w1029, w1033, w1034, w1035, w1037) -> (w1043:cluster{dbl[], "Waveform Read":dbl[]}[])
      }
      frame #1 {
        "Route Graph" <- w1060
      }
      frame #2 {
        n529 = Multiply(x=w1063, y=2) -> (x*y=w1062:i32)
        n530 = Greater Than 0?(x=w1069) -> (x > 0?=w1068:bool)
        n531 = Add(x=w1062, y=w1061) -> (x+y=w1066:i32)
        n532 = Multiply(x=w1066, y=w1065) -> (x*y=w1064:dbl)
        n533 = Select(t=w1066, s=w1068, f=w1064) -> (s? t:f=w1067:dbl)
        n534 = property on="Route Graph" class="XYGraph (strict)"() -> ("XScale.Maximum"=w1071:dbl)  [unwired: 2 in, 2 out]
        n535 = Greater?(x=w1067, y=w1071) -> (0:w1070:bool)
        n536 = case shown="True" w1070 {
          tunnel: w1067 -> [_ w1073]
          frame False {
          }
          frame True {
            n537 = property on="Route Graph" class="XYGraph (strict)"("XScale.Maximum"=w1073) -> ()  [unwired: 2 in, 2 out]
          }
        }
      }
    }
    n538 = call "_nr_CheckRasterSettings.vi"("Begin Raster"=w141, "Pixel"=w288, "Line"=w287, "Frame"=w286) -> ("continue with scan"=w289:bool)  [unwired: 2 in, 9 out]
    n539 = Bundle("Pixel Route"=w314, "Line Route"=w313, "Frame Route"=w312) -> (w309:T38)  [unwired: 1 out]
    n540 = Unbundle By Name(w178) -> ("Pixel uses Waveform Acquisition IN"=w175:bool)
    n541 = Unbundle By Name(w224) -> ("Pixel uses Waveform Acquisition IN"=w177:bool)
    n542 = case shown="True" "SaveDeviceData" {
      tunnel: w415 -> [_ w1706]
      tunnel: w233 -> [_ _]
      tunnel: path "C:/" ("file (use dialog)") -> [_ w1704]
      frame False {
      }
      frame True {
        n543 = call "File Dialog"("start path"=w1704) -> ("selected path"=w1705:path, "cancelled"=w1703:bool)  [unwired: 6 in, 7 out]
        n544 = case shown="False" w1703 {
          tunnel: w1706 -> [w1708 _]
          tunnel: w1705 -> [w1707 _]
          frame False {
            n545 = Write to Text File(file (use dialog)=w1707, text=w1708) -> ()  [unwired: 1 in, 4 out]
          }
          frame True {
          }
        }
      }
    }
    n546 = case shown="True" "Ignore" {
      tunnel: " A Template has been selected\nwhich has disabled the A/D Rate  \ncontrol. \n\nThis is likely because the \nA/D Rate of scans belonging to    \nthis Template is effected by a      \ncombination of template-specific  \ndelays (such as when Raster       \nScanning).                                    " ("message") -> [_ w1460]
      frame False {
      }
      frame True {
        n547 = One Button Dialog(message=w1460) -> ()  [unwired: 2 out]
      }
    }
    n548 = control-ref of="Tab Control"() -> (w143:refnum<vi>)
    n549 = control-ref of="Begin Raster"() -> (w311:refnum<vi>)
    n550 = control-ref of="Est. R.S. time"() -> (w308:refnum<vi>)
    n551 = case shown="True" "Clear Graph" {
      tunnel: "Clear run history \nfrom graph?" ("message") -> [_ w1607]
      tunnel: [FALSE ("T button?") w1606] -> w389
      frame False {
      }
      frame True {
        n552 = Two Button Dialog(message=w1607) -> (T button?=w1606:bool)  [unwired: 2 out]
      }
    }
    n553 = Unbundle(w345) -> ("Template"=w168:u16, "Template"=w167:u16, "pulse template"=w165:bool)
    n554 = Or(x=w389, y=w281) -> (x .or. y?=w388:bool)
    n555 = call "_nr_RasterScan.vi"("Pixel uses Waveform Acquisition IN"=w177, "WaveAcq Setup"=w310, "Raster Axis Config."=w71, "Raster Routes"=w309, "Raster Delays"=w70, "Est. R.S. time (s)"=w308, "Begin Raster"=w311, "time_of_scan"=w130, "Estimated Raster Scan Time"=w307, "Mirror motion on return?"=w223, "Incoming Handle"=w156, "20bit"=w231, "Tab Control"=w143) -> ("Array Size"=w302:i32, "Raster Finished"=w306:bool, "Pixel Read Arrays"=w303:dbl[][], "Line Read Arrays"=w305:dbl[][], "Frame Read Arrays"=w304:dbl[][], "time_of_scan"=w129:timestamp[])  [unwired: 9 in]
    n556 = Bundle("Template"=w168, "Template"=w167) -> (w166:cluster{"Template":u16, "Template":u16})  [unwired: 1 out]
    n557 = case shown="False" w388 {
      tunnel: w279 -> [w1610 _]
      tunnel: [w1610 w1612] -> w387
      tunnel: w256 -> [w1609 _]
      tunnel: [w1609 w1612] -> w386
      tunnel: w278 -> [w1608 _]
      tunnel: [w1608 T14 {{[], []}, {[], []}, {[], []}} ("All Route Reads")] -> w255
      frame False {
      }
      frame True {
        w1612 = cluster{dbl[], "Waveform Read":dbl[]} {[], "Waveform Read"=[]} ("Read")
      }
    }
    n558 = Unbundle(w166) -> ("Template"=w344:u16, "Template"=w228:u16)
    n559 = Bundle(w74, "Read"=w387, w280, "Read"=w386) -> (w67:T39)  [unwired: 1 out]
    n560 = Unbundle(w67) -> (w298:T37)  [unwired: 3 out]
    n561 = Equal?(x=w228, y=w340) -> (x = y?=w341:bool)
    n562 = Not Equal?(x=w344, y=w340) -> (x != y?=w343:bool)
    n563 = call "_nr_GenRSImage.vi"("Frame"=w304, "Raster Scan Image"=w299, "Line"=w305, "Pixel"=w303, "Array Size"=w302, "Begin Raster?"=w289) -> ("New Raster Image"=w301:cluster{dbl[], dbl[], dbl[]})
    n564 = And(x=w343, y=w341) -> (x .and. y?=w342:bool)
    n565 = Or(x=w342, y="Load") -> (x .or. y?=w339:bool)
    n566 = case shown="True" w339 {
      tunnel: [FALSE w1314] -> w338
      tunnel: ["" w1313] -> w337
      frame False {
      }
      frame True {
        n567 = Read from Text File() -> (text=w1313:string, cancelled=w1315:bool)  [unwired: 1 in, 5 out]
        n568 = Not(x=w1315) -> (.not. x?=w1314:bool)
      }
    }
    n569 = Bundle("Pixel Read Arrays"=w303, "Line Read Arrays"=w305, "Frame Read Arrays"=w304) -> (w285:T40)  [unwired: 1 out]
    n570 = Not(x=w177) -> (.not. x?=w176:bool)
    n571 = And(x=w175, y=w176) -> (x .and. y?=w174:bool)
    n572 = property on="Image Graph" class="XYGraph (strict)"() -> ("Active Plot"=w400:u32)  [unwired: 2 in, 2 out]
    n573 = case shown="True" w177 {
      frame False {
      }
      frame True {
        w613 = u8 2 ("Disabled")
        n574 = property on="Est. R.S. time" class="DigNum (strict)"("Disabled"=w613) -> ()  [unwired: 2 in, 2 out]
        n575 = property on="Pixel delay" class="DigNum (strict)"("Disabled"=w613) -> ()  [unwired: 2 in, 2 out]
      }
    }
    n576 = case shown="True" w174 {
      frame False {
      }
      frame True {
        w511 = u8 0 ("Disabled")
        n577 = property on="Est. R.S. time" class="DigNum (strict)"("Disabled"=w511) -> ()  [unwired: 2 in, 2 out]
        n578 = property on="Pixel delay" class="DigNum (strict)"("Disabled"=w511) -> ()  [unwired: 2 in, 2 out]
      }
    }
    n579 = Bundle("Template"=w228, "pulse template"=w165) -> (w164:cluster{"Template":u16, "pulse template":bool})  [unwired: 1 out]
    n580 = Unbundle(w164) -> ("Template"=w163:u16)  [unwired: 1 out]
    n581 = Not Equal?(x="Active Plot", y=w400) -> (x != y?=w398:bool)
    n582 = case shown="True" w398 {
      tunnel: "Active Plot" -> [_ w1625]
      tunnel: "Interpolation?" -> [w1621 _]
      tunnel: "Legend Visible" -> [w1620 _]
      tunnel: "Visible?" -> [w1619 _]
      frame False {
        n583 = Boolean To (0,1)(Boolean=w1621) -> (0, 1=w1624:i16)
        n584 = property on="Image Graph" class="XYGraph (strict)"("Plot.Visible?"=w1619) -> ()  [unwired: 2 in, 2 out]
        n585 = Multiply(x=i16 2, y=w1624) -> (x*y=w1623:i16)
        n586 = property on="Image Graph" class="XYGraph (strict)"("Plot.Plot Interpolation"=w1623) -> ()  [unwired: 2 in, 2 out]
        n587 = property on="Image Graph" class="XYGraph (strict)"("Legend Visible"=w1620) -> ()  [unwired: 2 in, 2 out]
      }
      frame True {
        n588 = stacked-sequence {
          tunnel: w1625 -> [w1626 _ _]
          frame #0 {
            n589 = property on="Image Graph" class="XYGraph (strict)"("Active Plot"=w1626) -> ()  [unwired: 2 in, 2 out]
          }
          frame #1 {
            n590 = property on="Image Graph" class="XYGraph (strict)"() -> ("Plot.Plot Interpolation"=w1630:u8)  [unwired: 2 in, 2 out]
            n591 = property on="Image Graph" class="XYGraph (strict)"() -> ("Plot.Visible?"=w1631:bool)  [unwired: 2 in, 2 out]
            n592 = Number To Boolean Array(number=w1630) -> (Boolean array=w1629:bool[])
            n593 = Index Array(array=w1629, index=1) -> (element=w1627:bool)
            n594 = local write "Visible?"(w1631) -> ()
            n595 = local write "Interpolation?"(w1627) -> ()
          }
          frame #2 {
            n596 = property on="Image Graph" class="XYGraph (strict)"() -> ("Legend Visible"=w1632:bool)  [unwired: 2 in, 2 out]
            n597 = local write "Legend Visible"(w1632) -> ()
          }
        }
      }
    }
    n598 = flat-sequence {
      tunnel: w306 -> [w872]
      tunnel: w192 -> [w874]
      tunnel: w80 -> [w873]
      tunnel: w184 -> [w870]
      tunnel: w146 -> [w869]
      frame #0 {
        n599 = case shown="True" w872 {
          frame False {
          }
          frame True {
            w877 = TRUE  # fit graph once
            w879 = u8 4 items=["Point by Point", "Time in milliseconds", "Frame", "Line", "Pixel"] ("X-Axis Display")
            w880 = u8 3 items=["Point by Point", "Time in milliseconds", "Frame", "Line", "Pixel"] ("Y-Axis Display")
            w881 = u32 2 items=["Individual Route Scan", "Run All Routes Scan", "Raster Scan"] ("Now Showing")
            n600 = local write "fit graph once"(w877) -> ()
            n601 = local write "Now Showing"(w881) -> ()
            n602 = local write "X-Axis Display"(w879) -> ()
            n603 = local write "Y-Axis Display"(w880) -> ()
            n604 = local write "Tab Control"(T19."Build Graph Image" ("Tab Control")) -> ()
          }
        }
        n605 = local read "Adv ISS Control"() -> (w871:bool)
        n606 = Unbundle(w873) -> ("Incoming Handle"=w876:i32)  [unwired: 2 out]
        n607 = call "_nr_ISSprepost.vi"("Before Scan"=FALSE ("End:Aux"), "ISS pre-post Use Advanced"=w871, "ISS pre-post"=w874, "Handle"=w876, "ISS pre-post Advanced Config"=w870, "ISS Info"=w869, "Enable"=w872) -> ()  [unwired: 2 out]
      }
    }
    n608 = Unbundle(w67) -> (w336:T37, "Read"=w368:cluster{dbl[], "Waveform Read":dbl[]}, w364:cluster{dbl[], dbl[]}, "Read"=w369:cluster{dbl[], "Waveform Read":dbl[]})
    n609 = Not Equal?(x=w259, y=u16 10) -> (x != y?=w273:bool)
    n610 = flat-sequence {
      tunnel: "AddPath" -> [w1082]
      tunnel: w260 -> [w1081]
      tunnel: w259 -> [w1080]
      tunnel: w273 -> [w1079]
      tunnel: w264 -> [w1078]
      tunnel: w272 -> [w1077]
      tunnel: "DeletePath" -> [w1076]
      tunnel: w270 -> [w1075]
      tunnel: [w1074] -> w269
      frame #0 {
        # "ADD / DELETE PATH"
        n611 = control-ref of="Current #:"() -> (w1088:refnum<vi>)
        n612 = control-ref of="Paths in X Route:"() -> (w1086:refnum<vi>)
        n613 = control-ref of="Paths in Y Route:"() -> (w1085:refnum<vi>)
        n614 = control-ref of="Paths in Z Route:"() -> (w1084:refnum<vi>)
        n615 = control-ref of="Axis"() -> (w1087:refnum<vi>)
        n616 = Bundle("Current #:"=w1088, "Axis"=w1087, "Paths in X Route:"=w1086, "Paths in Y Route:"=w1085, "Paths in Z Route:"=w1084) -> (w1083:T41)  [unwired: 1 out]
        n617 = call "_nr_AddDeletePath.vi"("Current #:"=w1081, "AddPath"=w1082, "AddDeletePath References"=w1083, "Path Type"=w1080, "Valid Path Type"=w1079, "function array"=w1078, "Current Route"=w1077, "DeletePath"=w1076, "Paths in Z Route:"=w1075) -> ("New Route"=w1074:cluster{dbl[], dbl[], i32[], u16[]})  [unwired: 6 out]
      }
    }
    n618 = flat-sequence {
      tunnel: w369 -> [w901]
      tunnel: w368 -> [w897]
      tunnel: w367 -> [w896]
      tunnel: [w892] -> w363
      tunnel: [w891] -> w335
      tunnel: w154 -> [w890]
      tunnel: w81 -> [w889]
      frame #0 {
        # "INSERT NEW READ IMAGE"
        n619 = Unbundle(w889) -> ("Axis"=w888:u32)  [unwired: 2 out]
        n620 = Unbundle(w890) -> ("Read"=w898:cluster{dbl[], "Waveform Read":dbl[]}, "Read"=w900:cluster{dbl[], "Waveform Read":dbl[]}, "Read"=w899:cluster{dbl[], "Waveform Read":dbl[]})
        n621 = Unbundle(w896) -> ("Read"=w895:cluster{dbl[], "Waveform Read":dbl[]}, "Read"=w894:cluster{dbl[], "Waveform Read":dbl[]}, "Read"=w893:cluster{dbl[], "Waveform Read":dbl[]})
        n622 = case shown="1, Default" w888 {
          tunnel: w897 -> [w905 w908 w912]
          tunnel: [w903 w909 w913] -> w891
          tunnel: w894 -> [_ w907 w911]
          tunnel: w893 -> [w904 _ w910]
          tunnel: w895 -> [w902 w906 _]
          frame 2 {
            n623 = Bundle("Read"=w902, "Read"=w905, "Read"=w904) -> (w903:T12)  [unwired: 1 out]
          }
          frame 3 {
            n624 = Bundle("Read"=w906, "Read"=w907, "Read"=w908) -> (w909:T12)  [unwired: 1 out]
          }
          frame 1, Default {
            n625 = Bundle("Read"=w912, "Read"=w911, "Read"=w910) -> (w913:T12)  [unwired: 1 out]
          }
        }
        n626 = case shown="1, Default" w888 {
          tunnel: w901 -> [w917 w920 w924]
          tunnel: [w915 w921 w925] -> w892
          tunnel: w900 -> [_ w919 w923]
          tunnel: w899 -> [w916 _ w922]
          tunnel: w898 -> [w914 w918 _]
          frame 2 {
            n627 = Bundle("Read"=w914, "Read"=w917, "Read"=w916) -> (w915:T12)  [unwired: 1 out]
          }
          frame 3 {
            n628 = Bundle("Read"=w918, "Read"=w919, "Read"=w920) -> (w921:T12)  [unwired: 1 out]
          }
          frame 1, Default {
            n629 = Bundle("Read"=w924, "Read"=w923, "Read"=w922) -> (w925:T12)  [unwired: 1 out]
          }
        }
      }
    }
    n630 = Unbundle(w269) -> (w403:i32[])  [unwired: 3 out]
    n631 = Array Size(array=w403) -> (size(s)=w404:i32)
    n632 = for {
      N: w404 -> [_]
      tunnel: w403 -> [w1633] mode=indexing
      shift-right: [w1635] -> w402
      shift-left: 0 -> [w1634]
      n633 = Add(x=w1633, y=w1634) -> (x+y=w1635:i32)
    }
    n634 = local read "Path Type"() -> (w230:u16)
    n635 = Multiply(x=w179, y=w402) -> (x*y=→"Time to Command Route (ms):":dbl)
    n636 = case shown="2" w230 {
      tunnel: [u8 2 ("Disabled") u8 2 ("Disabled") u8 0 ("Disabled") u8 0 ("Disabled") u8 0 ("Disabled") u8 0 ("Disabled")] -> w229
      frame 0 {
      }
      frame 1 {
      }
      frame 2 {
      }
      frame 3 {
      }
      frame 4 {
      }
      frame 5, Default {
      }
    }
    n637 = property on="function:" class="Str"("Disabled"=w229) -> ()  [unwired: 2 in, 2 out]
    n638 = flat-sequence {
      tunnel: w277 -> [w1177]
      tunnel: w269 -> [w1174]
      tunnel: [w1171] -> w256
      tunnel: [w1170] -> w284
      tunnel: "Current #:" -> [w1169]
      tunnel: w270 -> [w1168]
      frame #0 {
        # "COPY, PASTE, OR RESET ROUTE"
        n639 = control-ref of="Saved Route"() -> (w1183:refnum<vi>)
        n640 = control-ref of="Current #:"() -> (w1181:refnum<vi>)
        n641 = control-ref of="Paths in X Route:"() -> (w1180:refnum<vi>)
        n642 = control-ref of="Paths in Y Route:"() -> (w1179:refnum<vi>)
        n643 = control-ref of="Paths in Z Route:"() -> (w1178:refnum<vi>)
        n644 = control-ref of="Axis"() -> (w1182:refnum<vi>)
        n645 = Bundle("Saved Route"=w1183, "Axis"=w1182, "Current #:"=w1181, "Paths in X Route:"=w1180, "Paths in Y Route:"=w1179, "Paths in Z Route:"=w1178) -> (w1172:T42)  [unwired: 1 out]
        n646 = call "_nr_CopyPasteReset.vi"("Reset"="Reset", "Current Route"=w1174, "Read"=w1177, "Save Route"="Save Route", "Load Route"="Load Route", "Current #:"=w1169, "Paths in Route:"=w1168, "Copy/Paste/Reset References"=w1172) -> ("Read"=w1171:cluster{dbl[], "Waveform Read":dbl[]}, "New Route"=w1170:cluster{dbl[], dbl[], i32[], u16[]})  [unwired: 6 out]
      }
    }
    n647 = Equal?(x=T16."ISS Config." ("Tab Control"), y="Tab Control") -> (x = y?=w333:bool)
    n648 = case shown="True" w333 {
      tunnel: w146 -> [w1226 w1275]
      tunnel: [w1226 w1271] -> w227
      tunnel: w334 -> [_ w1240]
      frame False {
        (unwired) FALSE ("x .or. y?")
      }
      frame True {
        n649 = case shown="True" "PulsePix" {
          tunnel: w1240 -> [_ w1282]
          frame False {
          }
          frame True {
            n650 = dll-call lib="C:/Users/Labview/Desktop/64-bit VIs/Madlib.dll" fn="MCL_PixelClock"("handle"=w1282) -> ()  [unwired: 4 in, 3 out]
          }
        }
        n651 = case shown="True" "PulseLine" {
          tunnel: w1240 -> [_ w1281]
          frame False {
          }
          frame True {
            n652 = dll-call lib="C:/Users/Labview/Desktop/64-bit VIs/Madlib.dll" fn="MCL_LineClock"("handle"=w1281) -> ()  [unwired: 4 in, 3 out]
          }
        }
        n653 = case shown="True" "PulseFrame" {
          tunnel: w1240 -> [_ w1280]
          frame False {
          }
          frame True {
            n654 = dll-call lib="C:/Users/Labview/Desktop/64-bit VIs/Madlib.dll" fn="MCL_FrameClock"("handle"=w1280) -> ()  [unwired: 4 in, 3 out]
          }
        }
        n655 = case shown="True" "PulseAux" {
          tunnel: w1240 -> [_ w1279]
          frame False {
          }
          frame True {
            n656 = dll-call lib="C:/Users/Labview/Desktop/64-bit VIs/Madlib.dll" fn="MCL_AuxClock"("handle"=w1279) -> ()  [unwired: 4 in, 3 out]
          }
        }
        n657 = call "_nr_ISS_confirmOptions.vi"("PixBindAxis"="PixBindAxis", "LineBindAxis"="LineBindAxis", "FrameBindAxis"="FrameBindAxis", "AuxBindAxis"="AuxBindAxis") -> ("PixBindAxis (out)"=w1235:T4, "LineBindAxis (out)"=w1234:T4, "ISS Choices are Valid"=w1250:bool, "FrameBindAxis  (out)"=w1233:T4, "AuxBindAxis  (out)"=w1232:T4)  [unwired: 7 out]
        n658 = And(x=w1250, y="ISSConfirm") -> (x .and. y?=w1254:bool)
        n659 = Select(t=u8 0 ("Disabled"), s=w1250, f=u8 2) -> (s? t:f=w1251:u8)
        n660 = property on="ISSConfirm" class="Bool"("Disabled"=w1251) -> ()  [unwired: 2 in, 2 out]
        n661 = case shown="True" "ISSReset" {
          tunnel: w1240 -> [_ w1301]
          tunnel: w1254 -> [w1299 w1300]
          tunnel: [w1299 w1300] -> w1259
          frame False {
          }
          frame True {
            n662 = stacked-sequence {
              tunnel: w1301 -> [w1302 w1306 w1310]
              frame #0 {
                # "IssReset"
                n663 = dll-call lib="C:/Users/Labview/Desktop/64-bit VIs/Madlib.dll" fn="MCL_IssResetDefaults"("handle"=w1302) -> ()  [unwired: 4 in, 3 out]
              }
              frame #1 {
                # "unbind WR"
                n664 = dll-call lib="C:/Users/Labview/Desktop/64-bit VIs/Madlib.dll" fn="MCL_IssBindClockToAxis"("clock (1=Pixel)"=1, "mode (2=Low to High)"=4, "axis (1=X)"=5, "handle"=w1306) -> ()  [unwired: 7 in, 3 out]
              }
              frame #2 {
                # "undbind WW"
                n665 = dll-call lib="C:/Users/Labview/Desktop/64-bit VIs/Madlib.dll" fn="MCL_IssBindClockToAxis"("clock (1=Pixel)"=2, "mode (2=Low to High)"=4, "axis (1=X)"=6, "handle"=w1310) -> ()  [unwired: 7 in, 3 out]
              }
            }
          }
        }
        n666 = Unbundle(w1275) -> ("ISSReset"=w1245:bool, "ISS Confirmed Options"=w1246:T29, "ISS Confirmed Options"=w1247:T29, "ISS Confirmed Options"=w1248:T29, "ISS Confirmed Options"=w1249:T29)
        n667 = call "_nr_ISS.vi"("Polarity"="FramePol", "clock (1=Pixel)"=3, "Reset"="ISSReset", "Pulse"="FramePulse", "Axis Binding"=w1233, "ISS Confirmed Options (Feedback)"=w1248, "Confirm"=w1259, "Incoming Handle"=w1240) -> ("ISS Confirmed Options"=w1256:T29)  [unwired: 2 in, 5 out]
        n668 = call "_nr_ISS.vi"("Polarity"="PixPol", "clock (1=Pixel)"=1, "Reset"="ISSReset", "Pulse"="PixPulse", "Axis Binding"=w1235, "ISS Confirmed Options (Feedback)"=w1246, "Confirm"=w1259, "Incoming Handle"=w1240) -> ("ISS Confirmed Options"=w1272:T29)  [unwired: 2 in, 5 out]
        n669 = call "_nr_ISS.vi"("Polarity"="LinePol", "clock (1=Pixel)"=2, "Reset"="ISSReset", "Pulse"="LinePulse", "Axis Binding"=w1234, "ISS Confirmed Options (Feedback)"=w1247, "Confirm"=w1259, "Incoming Handle"=w1240) -> ("ISS Confirmed Options"=w1267:T29)  [unwired: 2 in, 5 out]
        n670 = call "_nr_ISS.vi"("Polarity"="AuxPol", "clock (1=Pixel)"=4, "Reset"="ISSReset", "Pulse"="AuxPulse", "Axis Binding"=w1232, "ISS Confirmed Options (Feedback)"=w1249, "Confirm"=w1259, "Incoming Handle"=w1240) -> ("ISS Confirmed Options"=w1255:T29)  [unwired: 2 in, 5 out]
        n671 = Or(x="PixRestore", y=w1245) -> (x .or. y?=w1231:bool)
        n672 = Or(x=w1245, y="LineRestore") -> (x .or. y?=w1230:bool)
        n673 = Or(x="FrameRestore", y=w1245) -> (x .or. y?=w1229:bool)
        n674 = Or(x="AuxRestore", y=w1245) -> (x .or. y?=w1228:bool)
        n675 = case shown="True" w1231 {
          tunnel: w1272 -> [_ w1298]
          frame False {
          }
          frame True {
            n676 = Unbundle(w1298) -> ("Pixel Polarity"=w1297:enum16{"Low", "High"}, "Pixel Pulse"=w1296:enum16{"Low to High", "High to Low"}, "Pixel Bind"=w1295:T4)  [unwired: 1 out]
            n677 = local write "PixPulse"(w1296) -> ()
            n678 = local write "PixPol"(w1297) -> ()
            n679 = local write "PixBindAxis"(w1295) -> ()
          }
        }
        n680 = case shown="True" w1230 {
          tunnel: w1267 -> [_ w1294]
          frame False {
          }
          frame True {
            n681 = Unbundle(w1294) -> ("Pixel Polarity"=w1291:enum16{"Low", "High"}, "Pixel Pulse"=w1292:enum16{"Low to High", "High to Low"}, "Pixel Bind"=w1293:T4)  [unwired: 1 out]
            n682 = local write "LinePulse"(w1292) -> ()
            n683 = local write "LinePol"(w1291) -> ()
            n684 = local write "LineBindAxis"(w1293) -> ()
          }
        }
        n685 = case shown="True" w1229 {
          tunnel: w1256 -> [_ w1290]
          frame False {
          }
          frame True {
            n686 = Unbundle(w1290) -> ("Pixel Polarity"=w1289:enum16{"Low", "High"}, "Pixel Pulse"=w1288:enum16{"Low to High", "High to Low"}, "Pixel Bind"=w1287:T4)  [unwired: 1 out]
            n687 = local write "FramePulse"(w1288) -> ()
            n688 = local write "FrameBindAxis"(w1287) -> ()
            n689 = local write "FramePol"(w1289) -> ()
          }
        }
        n690 = case shown="True" w1228 {
          tunnel: w1255 -> [_ w1286]
          frame False {
          }
          frame True {
            n691 = Unbundle(w1286) -> ("Pixel Polarity"=w1285:enum16{"Low", "High"}, "Pixel Pulse"=w1284:enum16{"Low to High", "High to Low"}, "Pixel Bind"=w1283:T4)  [unwired: 1 out]
            n692 = local write "AuxPulse"(w1284) -> ()
            n693 = local write "AuxBindAxis"(w1283) -> ()
            n694 = local write "AuxPol"(w1285) -> ()
          }
        }
        n695 = Bundle("ISSReset"="ISSReset", "ISS Confirmed Options"=w1272, "ISS Confirmed Options"=w1267, "ISS Confirmed Options"=w1256, "ISS Confirmed Options"=w1255) -> (w1271:T9)  [unwired: 1 out]
      }
    }
    n696 = flat-sequence {
      tunnel: w284 -> [w1166]
      tunnel: w76 -> [w1165]
      tunnel: w283 -> [w1164]
      tunnel: w267 -> [w1163]
      tunnel: w179 -> [w1162]
      tunnel: w282 -> [w1161]
      tunnel: [w1160] -> w110
      tunnel: [w1159] -> w281
      tunnel: [w1158] -> w81
      tunnel: w72 -> [w1157]
      frame #0 {
        # "UPDATE ROUTE"
        n697 = control-ref of="Current #:"() -> (w1167:refnum<vi>)
        n698 = call "_nr_UpdateRoute.vi"("Axis"=w1157, "New Route"=w1166, "Incoming Handle"=w1165, "Previous Axis"=w1164, "Existing Routes"=w1163, "A/D Rate\n16-bit 2"=w1162, "Current #:"=w1167, "A/D Rate\n16-bit 3"=w1161) -> ("New Routes"=w1160:T21, "A/D Rate Changed"=w1159:bool, "Axis Info"=w1158:T7)  [unwired: 9 out]
      }
    }
    n699 = Not(x=w274) -> (.not. x?=w151:bool)
    n700 = Not Equal To 0?(x=w276) -> (x != 0?=w376:bool)
    n701 = property on="Tab Control" class="TabCtl (strict)"("Tabs Visible?"=w151) -> ()  [unwired: 2 in, 2 out]
    n702 = Bundle("message"="The A/D rate must be equal to, or greater than,2ms per point when not using Wave Acquisition. Correct this error and try again", "message"="When performing WaveForm\nAcquisition the A/D rate cannot\nexceed 5ms. Correct this error\nand retry.") -> (w93:cluster{"message":string, "message":string})  [unwired: 1 out]
    n703 = Bundle("string"="This is an unidentified error.", "string"="This error has been identified as MCL_GENERAL_ERROR; \nan error occuring due to an internal sanity check failing.", "string"="This error has been identified as MCL_DEV_ERROR; a  \nproblem occurred when transfering data to the Nano-\nDrive. It is likely that the Nano-Drive will Have to be \npower cycled to correct these problems.", "string"="This error has been identified as MCL_DEV_NOT_ATTACHED;  \nThe Nano-Drive cannot complete the task because \nit is not attached.", "string"="This error has been identified as MCL_USAGE_ERROR; a \nfunction has been called from the libray which this Nano-\nDrive does not support.", "string"="This error has been identified as MCL_DEV_NOT_READY;\nThe Nano-Drive is currently completing, or waiting to \ncomplete, a task.", "string"="This error has been identified as MCL_ARGUMENT_ERROR;\nan argument is out of range or a required pointer is equal \nto NULL.", "string"="This error has been identified as MCL_INVALID_AXIS;\nattempting an operation on an axis that does not exist\nin the Nano-Drive.", "string"="This error has been identified as MCL_INVALID_HANDLE;\nthe handle was not valid for this instance of the DLL.") -> (w98:T43)  [unwired: 1 out]
    n704 = case shown="False" w376 {
      tunnel: w276 -> [_ w1504]
      tunnel: "The Madlib.dll file used during this scan has returned an error \ncode. An error report may be available via the Details button." ("message") -> [_ w1507]
      tunnel: "The following error has occured:   " ("string") -> [_ w1503]
      tunnel: w98 -> [_ w1502]
      tunnel: w274 -> [w1492 _]
      tunnel: w93 -> [_ w1501]
      tunnel: w72 -> [w1491 _]
      frame False {
        # "No error during\nrecent run?"
        n705 = case shown="True" w1492 {
          tunnel: w1491 -> [_ w1493]
          frame False {
          }
          frame True {
            n706 = flat-sequence {
              tunnel: w1493 -> [w1495]
              frame #0 {
                w1496 = u32 0 items=["Individual Route Scan", "Run All Routes Scan", "Raster Scan"] ("Now Showing")
                w1499 = u8 1 items=["Point by Point", "Time in milliseconds", "Axis: X Position", "Axis: Y Position", "Axis: Z Position"] ("X-Axis Display")
                n707 = Add(x=w1495, y=u32 1) -> (x+y=w1498:u32)
                n708 = local write "X-Axis Display"(w1499) -> ()
                n709 = local write "Y-Axis Display"(w1498) -> ()
                n710 = local write "Now Showing"(w1496) -> ()
                n711 = local write "Tab Control"(T19."Build Graph Image" ("Tab Control")) -> ()
              }
              frame #1 {
                w1500 = TRUE  # fit graph once
                "fit graph once" <- w1500
              }
            }
          }
        }
      }
      frame True {
        n712 = Two Button Dialog(message=w1507, 1:"Details" ("F button name (\"Cancel\")")) -> (T button?=w1505:bool)  [unwired: 1 out]
        n713 = case shown="False" w1505 {
          tunnel: w1504 -> [w1511 _]
          tunnel: w1503 -> [w1510 _]
          tunnel: w1502 -> [w1509 _]
          tunnel: w1501 -> [w1508 _]
          frame False {
            n714 = case shown="-2" w1511 {
              tunnel: w1511 -> [w1518 w1525 w1532 w1539 w1546 w1553 w1560 w1567 w1574 w1581 w1588]
              tunnel: w1510 -> [w1517 w1524 w1531 w1538 w1545 w1552 w1559 w1566 w1573 w1580 w1587]
              tunnel: w1509 -> [w1513 w1520 w1527 w1534 w1541 w1548 w1555 w1562 w1569 _ _]
              tunnel: w1508 -> [_ _ _ _ _ _ _ _ _ w1576 w1583]
              frame 0, Default {
                n715 = Number To Decimal String(number=w1518) -> (decimal integer string=w1516:string)  [unwired: 1 out]
                n716 = Unbundle(w1513) -> ("string"=w1512:string)  [unwired: 8 out]
                n717 = Concatenate Strings(w1517, w1516, "\r", w1512) -> (w1514:string)
                n718 = One Button Dialog(message=w1514) -> ()  [unwired: 2 out]
              }
              frame -1 {
                n719 = Number To Decimal String(number=w1525) -> (decimal integer string=w1523:string)  [unwired: 1 out]
                n720 = Unbundle(w1520) -> ("string"=w1519:string)  [unwired: 8 out]
                n721 = Concatenate Strings(w1524, w1523, "\r", w1519) -> (w1521:string)
                n722 = One Button Dialog(message=w1521) -> ()  [unwired: 2 out]
              }
              frame -2 {
                n723 = Number To Decimal String(number=w1532) -> (decimal integer string=w1530:string)  [unwired: 1 out]
                n724 = Unbundle(w1527) -> ("string"=w1526:string)  [unwired: 8 out]
                n725 = Concatenate Strings(w1531, w1530, "\r", w1526) -> (w1528:string)
                n726 = One Button Dialog(message=w1528) -> ()  [unwired: 2 out]
              }
              frame -3 {
                n727 = Number To Decimal String(number=w1539) -> (decimal integer string=w1537:string)  [unwired: 1 out]
                n728 = Unbundle(w1534) -> ("string"=w1533:string)  [unwired: 8 out]
                n729 = Concatenate Strings(w1538, w1537, "\r", w1533) -> (w1535:string)
                n730 = One Button Dialog(message=w1535) -> ()  [unwired: 2 out]
              }
              frame -4 {
                n731 = Number To Decimal String(number=w1546) -> (decimal integer string=w1544:string)  [unwired: 1 out]
                n732 = Unbundle(w1541) -> ("string"=w1540:string)  [unwired: 8 out]
                n733 = Concatenate Strings(w1545, w1544, "\r", w1540) -> (w1542:string)
                n734 = One Button Dialog(message=w1542) -> ()  [unwired: 2 out]
              }
              frame -5 {
                n735 = Number To Decimal String(number=w1553) -> (decimal integer string=w1551:string)  [unwired: 1 out]
                n736 = Unbundle(w1548) -> ("string"=w1547:string)  [unwired: 8 out]
                n737 = Concatenate Strings(w1552, w1551, "\r", w1547) -> (w1549:string)
                n738 = One Button Dialog(message=w1549) -> ()  [unwired: 2 out]
              }
              frame -6 {
                n739 = Number To Decimal String(number=w1560) -> (decimal integer string=w1558:string)  [unwired: 1 out]
                n740 = Unbundle(w1555) -> ("string"=w1554:string)  [unwired: 8 out]
                n741 = Concatenate Strings(w1559, w1558, "\r", w1554) -> (w1556:string)
                n742 = One Button Dialog(message=w1556) -> ()  [unwired: 2 out]
              }
              frame -7 {
                n743 = Number To Decimal String(number=w1567) -> (decimal integer string=w1565:string)  [unwired: 1 out]
                n744 = Unbundle(w1562) -> ("string"=w1561:string)  [unwired: 8 out]
                n745 = Concatenate Strings(w1566, w1565, "\r", w1561) -> (w1563:string)
                n746 = One Button Dialog(message=w1563) -> ()  [unwired: 2 out]
              }
              frame -8 {
                n747 = Number To Decimal String(number=w1574) -> (decimal integer string=w1572:string)  [unwired: 1 out]
                n748 = Unbundle(w1569) -> ("string"=w1568:string)  [unwired: 8 out]
                n749 = Concatenate Strings(w1573, w1572, "\r", w1568) -> (w1570:string)
                n750 = One Button Dialog(message=w1570) -> ()  [unwired: 2 out]
              }
              frame -9 {
                n751 = Number To Decimal String(number=w1581) -> (decimal integer string=w1579:string)  [unwired: 1 out]
                n752 = Unbundle(w1576) -> ("message"=w1575:string)  [unwired: 1 out]
                n753 = Concatenate Strings(w1580, w1579, "\r", w1575) -> (w1577:string)
                n754 = One Button Dialog(message=w1577) -> ()  [unwired: 2 out]
              }
              frame -10 {
                n755 = Number To Decimal String(number=w1588) -> (decimal integer string=w1586:string)  [unwired: 1 out]
                n756 = Unbundle(w1583) -> ("message"=w1582:string)  [unwired: 1 out]
                n757 = Concatenate Strings(w1587, w1586, "\r", w1582) -> (w1584:string)
                n758 = One Button Dialog(message=w1584) -> ()  [unwired: 2 out]
              }
            }
          }
          frame True {
          }
        }
      }
    }
    n759 = Unbundle(w110) -> ("Z"=w362:cluster{dbl[], dbl[], i32[], u16[]}, "Y"=w361:cluster{dbl[], dbl[], i32[], u16[]}, "X"=w360:cluster{dbl[], dbl[], i32[], u16[]})
    n760 = case shown="True" "SAVE" {
      tunnel: [w1432 w1459] -> _
      tunnel: w87 -> [w1432 w1459]
      tunnel: [w1431 w1458] -> w89
      tunnel: w301 -> [w1431 w1458]
      tunnel: [w1430 w1457] -> w83
      tunnel: w255 -> [w1430 w1457]
      tunnel: [w1429 w1456] -> w138
      tunnel: w365 -> [w1429 w1456]
      tunnel: [w1428 w1455] -> _
      tunnel: w336 -> [w1428 w1455]
      tunnel: [w1427 w1454] -> w137
      tunnel: w335 -> [w1427 w1454]
      tunnel: [w1426 w1453] -> w136
      tunnel: w364 -> [w1426 w1453]
      tunnel: [w1425 w1452] -> w135
      tunnel: w363 -> [w1425 w1452]
      tunnel: [w1424 w1434] -> w352
      tunnel: w362 -> [w1424 w1434]
      tunnel: [w1423 w1433] -> w134
      tunnel: w361 -> [w1423 w1433]
      tunnel: [w1422 w1451] -> w353
      tunnel: w360 -> [w1422 w1451]
      tunnel: [w1421 w1450] -> w354
      tunnel: w334 -> [w1421 w1450]
      tunnel: [w1420 w1449] -> w355
      tunnel: w359 -> [w1420 w1449]
      tunnel: [w1419 w1448] -> w356
      tunnel: w358 -> [w1419 w1448]
      tunnel: [w1418 w1445] -> w357
      tunnel: w285 -> [w1418 w1445]
      tunnel: w179 -> [_ w1446]
      tunnel: w224 -> [w1417 w1444]
      tunnel: [w1417 w1444] -> w139
      tunnel: w163 -> [_ w1440]
      tunnel: w227 -> [w1416 w1439]
      tunnel: [w1416 w1439] -> w225
      tunnel: w222 -> [_ w1438]
      tunnel: [_ w1437] -> w140
      frame False {
      }
      frame True {
        n761 = local read "Paths in X Route:"() -> (w1443:u16)
        n762 = local read "Paths in Y Route:"() -> (w1442:u16)
        n763 = local read "Paths in Z Route:"() -> (w1441:u16)
        n764 = Bundle("Z"=w1434, "Y"=w1433, "X"=w1451, "Incoming Handle"=w1450, "Axis"=w1449, "A/D Rate\n16-bit 2"=w1448, "A/D Rate\n16-bit"=w1446, "Paths in X Route:"=w1443, "Paths in Y Route:"=w1442, "Paths in Z Route:"=w1441, "Template"=w1440, w1439, w1438) -> (w1437:T44)  [unwired: 1 out]
        n765 = To Variant(anything=w1437) -> (Variant=w1436:variant)
        n766 = Variant To Flattened String(Variant=w1436) -> (data string=w1447:string, 1:→"Type Descriptor":i16[])
        n767 = Write to Text File(text=w1447) -> ()  [unwired: 1 in, 5 out]
      }
    }
    n768 = case shown="True" w338 {
      tunnel: [w1323 w1347] -> w351
      tunnel: w352 -> [w1323 _]
      tunnel: [w1322 w1324] -> w350
      tunnel: w134 -> [w1322 _]
      tunnel: [w1321 w1348] -> w349
      tunnel: w353 -> [w1321 _]
      tunnel: w354 -> [w1317 w1334]
      tunnel: [w1320 w1349] -> w348
      tunnel: w355 -> [w1320 _]
      tunnel: [w1319 w1350] -> w347
      tunnel: w356 -> [w1319 _]
      tunnel: [w1318 w1326] -> _
      tunnel: w357 -> [w1318 w1326]
      tunnel: w261 -> [_ w1346]
      tunnel: [w1317 w1334] -> _
      tunnel: w337 -> [_ w1344]
      tunnel: [w1316 w1327] -> w226
      tunnel: w225 -> [w1316 _]
      tunnel: w140 -> [_ w1329]
      frame False {
      }
      frame True {
        w1325 = u16 0  # Current #:
        n769 = flat-sequence {
          tunnel: w1344 -> [w1355]
          tunnel: w1329 -> [w1353]
          tunnel: [w1352] -> w1328
          tunnel: [w1363] -> w1347
          tunnel: [w1364] -> w1324
          tunnel: [w1365] -> w1348
          tunnel: [w1366] -> w1349
          tunnel: [w1367] -> w1350
          tunnel: [w1362] -> w1345
          tunnel: [w1361] -> w1343
          tunnel: [w1360] -> w1342
          tunnel: [w1359] -> w1341
          tunnel: [w1358] -> w1340
          tunnel: [w1357] -> w1327
          tunnel: [w1356] -> w1333
          tunnel: w1328 -> [w1368]
          frame #0 {
            w1351 = i16[] [1632, 80, 13, 80, 16464, 4, 14, 64, 1, -1, -1, 4, 10, 20, 64, 1, -1, -1, 10, 16394, 1064, 30061, 10496, 14, 64, 1, -1, -1, 4, 3, 24, 64, 1, -1, -1, 14, 16390, 2131, 15664, 8202, 21053, 12544, 346, 80, 16464, 4, 14, 64, 1, -1, -1, 4, 10, 20, 64, 1, -1, -1, 10, 16394, 1064, 30061, 10496, 14, 64, 1, -1, -1, 4, 3, 24, 64, 1, -1, -1, 14, 16390, 2131, 15664, 8202, 21053, 12544, 345, 80, 16464, 4, 14, 64, 1, -1, -1, 4, 10, 20, 64, 1, -1, -1, 10, 16394, 1064, 30061, 10496, 14, 64, 1, -1, -1, 4, 3, 24, 64, 1, -1, -1, 14, 16390, 2131, 15664, 8202, 21053, 12544, 344, 20, 16387, 3913, 28259, 28525, 26990, 26400, 18529, 28260, 27749, 10, 16391, 1089, 30825, 29440, 22, 16394, 4417, 12100, 8274, 24948, 25866, 12598, 11618, 26996, 8242, 20, 16394, 3905, 12100, 8274, 24948, 25866, 12598, 11618, 26996, 22, 16390, 4432, 24948, 26739, 8297, 28192, 22560, 21103, 30068, 25914, 22, 16390, 4432, 24948, 26739, 8297, 28192, 22816, 21103, 30068, 25914, 22, 16390, 4432, 24948, 26739, 8297, 28192, 23072, 21103, 30068, 25914, 14, 16390, 2132, 25965, 28780, 24948, 25856, 852, 80, 5, 14, 16417, 2121, 21331, 21093, 29541, 29696, 208, 16464, 4, 20, 16387, 3939, 27759, 25451, 8232, 12605, 20585, 30821, 27689, 32, 16406, 2, 844, 28535, 1096, 26983, 26624, 3664, 27000, 25964, 8272, 28524, 24946, 26996, 30976, 42, 16406, 2, 2892, 28535, 8308, 28448, 18537, 26472, 2888, 26983, 26656, 29807, 8268, 28535, 2896, 27000, 25964, 8272, 30060, 29541, 86, 16406, 7, 1877, 28258, 28533, 28260, 1624, 8257, 30825, 29446, 22816, 16760, 26995, 1626, 8257, 30825, 29448, 16757, 30825, 27745, 29305, 3415, 24950, 25958, 28530, 27936, 21093, 24932, 3671, 24950, 25958, 28530, 27936, 22386, 26996, 25856, 2640, 27000, 25964, 8258, 26990, 25600, 5449, 21331, 8259, 28526, 26217, 29293, 25956, 8271, 28788, 26991, 28275, 208, 16464, 4, 20, 16387, 3939, 27759, 25451, 8232, 12605, 20585, 30821, 27689, 32, 16406, 2, 844, 28535, 1096, 26983, 26624, 3664, 27000, 25964, 8272, 28524, 24946, 26996, 30976, 42, 16406, 2, 2892, 28535, 8308, 28448, 18537, 26472, 2888, 26983, 26656, 29807, 8268, 28535, 2896, 27000, 25964, 8272, 30060, 29541, 86, 16406, 7, 1877, 28258, 28533, 28260, 1624, 8257, 30825, 29446, 22816, 16760, 26995, 1626, 8257, 30825, 29448, 16757, 30825, 27745, 29305, 3415, 24950, 25958, 28530, 27936, 21093, 24932, 3671, 24950, 25958, 28530, 27936, 22386, 26996, 25856, 2640, 27000, 25964, 8258, 26990, 25600, 5449, 21331, 8259, 28526, 26217, 29293, 25956, 8271, 28788, 26991, 28275, 208, 16464, 4, 20, 16387, 3939, 27759, 25451, 8232, 12605, 20585, 30821, 27689, 32, 16406, 2, 844, 28535, 1096, 26983, 26624, 3664, 27000, 25964, 8272, 28524, 24946, 26996, 30976, 42, 16406, 2, 2892, 28535, 8308, 28448, 18537, 26472, 2888, 26983, 26656, 29807, 8268, 28535, 2896, 27000, 25964, 8272, 30060, 29541, 86, 16406, 7, 1877, 28258, 28533, 28260, 1624, 8257, 30825, 29446, 22816, 16760, 26995, 1626, 8257, 30825, 29448, 16757, 30825, 27745, 29305, 3415, 24950, 25958, 28530, 27936, 21093, 24932, 3671, 24950, 25958, 28530, 27936, 22386, 26996, 25856, 2640, 27000, 25964, 8258, 26990, 25600, 5449, 21331, 8259, 28526, 26217, 29293, 25956, 8271, 28788, 26991, 28275, 208, 16464, 4, 20, 16387, 3939, 27759, 25451, 8232, 12605, 20585, 30821, 27689, 32, 16406, 2, 844, 28535, 1096, 26983, 26624, 3664, 27000, 25964, 8272, 28524, 24946, 26996, 30976, 42, 16406, 2, 2892, 28535, 8308, 28448, 18537, 26472, 2888, 26983, 26656, 29807, 8268, 28535, 2896, 27000, 25964, 8272, 30060, 29541, 86, 16406, 7, 1877, 28258, 28533, 28260, 1624, 8257, 30825, 29446, 22816, 16760, 26995, 1626, 8257, 30825, 29448, 16757, 30825, 27745, 29305, 3415, 24950, 25958, 28530, 27936, 21093, 24932, 3671, 24950, 25958, 28530, 27936, 22386, 26996, 25856, 2640, 27000, 25964, 8258, 26990, 25600, 5449, 21331, 8259, 28526, 26217, 29293, 25956, 8271, 28788, 26991, 28275, 382, 80, 4, 30, 16417, 6221, 26994, 29295, 29216, 28015, 29801, 28526, 8303, 28192, 29285, 29813, 29294, 16128, 210, 16464, 6, 26, 16394, 5202, 24915, 25393, 13922, 26996, 21093, 24932, 21089, 29797, 8265, 19968, 26, 16394, 5458, 24915, 25393, 13922, 26996, 22386, 26996, 25938, 24948, 25888, 18766, 26, 16394, 5458, 24915, 25394, 12386, 26996, 22386, 26996, 25938, 24948, 25888, 18766, 26, 16394, 5202, 24915, 25394, 12386, 26996, 21093, 24932, 21089, 29797, 8265, 19968, 40, 16417, 8784, 27000, 25964, 8309, 29541, 29472, 22369, 30309, 26223, 29293, 8257, 25457, 30057, 29545, 29801, 28526, 8265, 19968, 26, 16391, 5202, 24915, 25393, 13922, 26996, 9071, 26194, 25953, 25715, 8265, 19968, 8274, 24947, 29797, 29216, 21347, 24942, 8257, 25718, 24942, 25445, 25632, 20336, 29801, 28526, 29472, 20309, 21504, 36, 80, 3, 10, 16391, 1360, 27000, 25964, 10, 16391, 1100, 26990, 25856, 10, 16391, 1350, 29281, 28005, 100, 80, 5, 16, 16391, 2896, 27000, 25964, 8292, 25964, 24953, 22, 16391, 4421, 28260, 8303, 26144, 19561, 28261, 8292, 25964, 24953, 24, 16391, 4947, 29793, 29300, 8303, 26144, 19561, 28261, 8292, 25964, 24953, 16, 16391, 2886, 29281, 28005, 8292, 25964, 24953, 16, 16391, 2896, 27000, 25964, 8292, 30565, 27756]  # Type Descriptor
            n770 = Flattened String To Variant(6:w1355, 7:w1351) -> (3:w1354:variant)  [unwired: 1 in, 1 out]
            n771 = Variant To Data(type=w1353, Variant=w1354) -> (data=w1352:T44)  [unwired: 1 in, 1 out]
          }
          frame #1 {
            n772 = Unbundle(w1368) -> ("Z"=w1363:cluster{dbl[], dbl[], i32[], u16[]}, "Y"=w1364:cluster{dbl[], dbl[], i32[], u16[]}, "X"=w1365:cluster{dbl[], dbl[], i32[], u16[]}, "Axis"=w1366:u32, "A/D Rate\n16-bit 2"=w1367:dbl, "A/D Rate\n16-bit"=w1362:dbl, "Paths in X Route:"=w1361:u16, "Paths in Y Route:"=w1360:u16, "Paths in Z Route:"=w1359:u16, "Template"=w1358:u16, w1357:T9, w1356:T34)  [unwired: 1 out]
          }
        }
        n773 = local write "Current #:"(w1325) -> ()
        n774 = local write "Paths in X Route:"(w1343) -> ()
        n775 = local write "Paths in Y Route:"(w1342) -> ()
        n776 = local write "Paths in Z Route:"(w1341) -> ()
        n777 = case shown="True" w1346 {
          tunnel: w1345 -> [w1414 w1415]
          frame False {
            n778 = local write "A/D Rate\n16-bit"(w1414) -> ()
          }
          frame True {
            n779 = local write "A/D Rate\n20-bit"(w1415) -> ()
          }
        }
        n780 = local write "Template"(w1340) -> ()
        n781 = Unbundle(w1327) -> ("ISS Confirmed Options"=w1339:T29, "ISS Confirmed Options"=w1338:T29, "ISS Confirmed Options"=w1337:T29, "ISS Confirmed Options"=w1336:T29)  [unwired: 1 out]
        n782 = Build Array(w1339, w1338, w1337, w1336) -> (w1335:T45)
        n783 = flat-sequence {
          tunnel: w1335 -> [w1372]
          tunnel: w1334 -> [w1371]
          tunnel: w1333 -> [w1370]
          tunnel: [w1370] -> w1332
          tunnel: [w1369] -> w1330
          tunnel: w1327 -> [w1369]
          tunnel: w1332 -> [w1402]
          tunnel: [w1402] -> w1331
          tunnel: w1330 -> [w1397]
          tunnel: w1331 -> [w1413]
          frame #0 {
            n784 = for {
              tunnel: w1372 -> [w1374] mode=indexing
              tunnel: w1371 -> [w1375]
              n785 = Unbundle(w1374) -> ("clock (1=Pixel)"=w1380:i32, "Pixel Polarity"=w1379:enum16{"Low", "High"}, "Pixel Pulse"=w1378:enum16{"Low to High", "High to Low"}, "Pixel Bind"=w1377:T4)
              n786 = call "_nr_ISS.vi"("Polarity"=w1379, "clock (1=Pixel)"=w1380, "Reset"=FALSE, "Pulse"=w1378, "Axis Binding"=w1377, "ISS Confirmed Options (Feedback)"=w1374, "Confirm"=TRUE, "Incoming Handle"=w1375) -> ()  [unwired: 2 in, 6 out]
            }
          }
          frame #1 {
            n787 = Unbundle(w1397) -> ("ISS Confirmed Options"=w1398:T29, "ISS Confirmed Options"=w1401:T29, "ISS Confirmed Options"=w1400:T29, "ISS Confirmed Options"=w1399:T29)  [unwired: 1 out]
            n788 = Unbundle(w1398) -> ("Pixel Bind"=w1387:T4)  [unwired: 3 out]
            n789 = Unbundle(w1401) -> ("Pixel Bind"=w1388:T4)  [unwired: 3 out]
            n790 = Unbundle(w1400) -> ("Pixel Bind"=w1389:T4)  [unwired: 3 out]
            n791 = Unbundle(w1399) -> ("Pixel Bind"=w1390:T4)  [unwired: 3 out]
            n792 = local write "FrameBindAxis"(w1389) -> ()
            n793 = local write "LineBindAxis"(w1388) -> ()
            n794 = local write "AuxBindAxis"(w1390) -> ()
            n795 = local write "PixBindAxis"(w1387) -> ()
            n796 = Unbundle(w1397) -> ("ISS Confirmed Options"=w1396:T29, "ISS Confirmed Options"=w1395:T29, "ISS Confirmed Options"=w1394:T29, "ISS Confirmed Options"=w1393:T29)  [unwired: 1 out]
            n797 = Unbundle(w1396) -> ("Pixel Polarity"=w1392:enum16{"Low", "High"}, "Pixel Pulse"=w1391:enum16{"Low to High", "High to Low"})  [unwired: 2 out]
            n798 = Unbundle(w1395) -> ("Pixel Polarity"=w1386:enum16{"Low", "High"}, "Pixel Pulse"=w1385:enum16{"Low to High", "High to Low"})  [unwired: 2 out]
            n799 = Unbundle(w1394) -> ("Pixel Polarity"=w1384:enum16{"Low", "High"}, "Pixel Pulse"=w1383:enum16{"Low to High", "High to Low"})  [unwired: 2 out]
            n800 = Unbundle(w1393) -> ("Pixel Polarity"=w1382:enum16{"Low", "High"}, "Pixel Pulse"=w1381:enum16{"Low to High", "High to Low"})  [unwired: 2 out]
            n801 = local write "LinePol"(w1386) -> ()
            n802 = local write "LinePulse"(w1385) -> ()
            n803 = local write "FramePol"(w1384) -> ()
            n804 = local write "FramePulse"(w1383) -> ()
            n805 = local write "PixPol"(w1392) -> ()
            n806 = local write "PixPulse"(w1391) -> ()
            n807 = local write "AuxPol"(w1382) -> ()
            n808 = local write "AuxPulse"(w1381) -> ()
          }
          frame #2 {
            n809 = Unbundle(w1413) -> ("Mirror motion on return?"=w1403:bool, "RasterAxisConfig"=w1411:cluster{"Pixel":u32, "Line":u32, "Frame":u32}, "RasterDelays"=w1412:T5)  [unwired: 1 out]
            n810 = Unbundle(w1411) -> ("Pixel"=w1404:u32, "Line"=w1405:u32, "Frame"=w1406:u32)
            n811 = Unbundle(w1412) -> ("Pixel delay"=w1407:u32, "End of Line delay"=w1408:u32, "Start of Line delay"=w1409:u32, "Frame delay"=w1410:u32)  [unwired: 1 out]
            n812 = local write "Mirror motion on return?"(w1403) -> ()
            n813 = local write "End of Line delay"(w1408) -> ()
            n814 = local write "Start of Line delay"(w1409) -> ()
            n815 = local write "Line"(w1405) -> ()
            n816 = local write "Pixel delay"(w1407) -> ()
            n817 = local write "Pixel"(w1404) -> ()
            n818 = local write "Frame"(w1406) -> ()
            n819 = local write "Frame delay"(w1410) -> ()
          }
        }
      }
    }
    "DeviceLoaded" <- w329
  }
  n820 = case shown="True" w6 {
    frame False {
    }
    frame True {
      n821 = flat-sequence {
        frame #0 {
          # "Stop Sequence"
          n822 = for {
            N: 20 -> [_]
            n823 = dll-call lib="C:/Users/Labview/Desktop/64-bit VIs/Madlib.dll" fn="MCL_ReleaseAllHandles"() -> ()  [unwired: 3 in, 3 out]
          }
        }
        frame #1 {
          n824 = control-ref of="stop"() -> (w1710:refnum<vi>)
          n825 = property on="Property Node" class="Bool (strict)"(reference=w1710, "Visible"=FALSE) -> ()  [unwired: 1 in, 2 out]
        }
        frame #2 {
          n826 = Stop(stop? (T)=TRUE) -> ()
        }
      }
    }
  }
  "Scanning Indicator" <- FALSE ("Scanning Indicator")
